vi "main 0.9.5.testing.vi"() -> ()   [LabVIEW 2020]
uses:
  subvi/Newport ESP301/Newport ESP301.lvlib
  subvi/sp_manip.llb/sp_manip_lib.lvlib
  subvi/sp_manip.llb/tcp_gateway.lvlib
  subvi/PHOIBOS/DEFINITIONS/DEF_dev_type.ctl
  subvi/PHOIBOS/DEFINITIONS/DEF_dev_state.ctl
  <vilib>/Utility/file.llb/Write Delimited Spreadsheet (DBL).vi
  <vilib>/Utility/file.llb/Read Delimited Spreadsheet (string).vi
  <vilib>/Analysis/NI_AALBase.lvlib
  <vilib>/Analysis/1siggen.llb/Ramp Pattern by Samples.vi
  <vilib>/DAQmx/create/channels.llb/DAQmx Create Channel (AI-Voltage-Basic).vi
  <vilib>/DAQmx/read.llb/DAQmx Read (Analog DBL 1Chan 1Samp).vi
panel:
  out "Pics L":i32
  out "Pics NL":i32
  out "Voltage":dbl format="%0.2f"
  out "sideimg 2":dbl[][](graph)
  in  "Frame trigger \n(High Performance and QE only)":u16
  in  "Operating mode\nHP & QE / HS & DiCam Pro":u32
  out "Waveform Chart":dbl(graph)
  out "G2 X":cluster{dbl[], "Ramp Pattern":dbl[]}(graph)={array[344 elements], "Ramp Pattern"=[5593.0, 5541.0, 5578.0, 5573.0, 5542.0, 5582.0, 5523.0, 5570.0, 5578.0, 5560.0, 5581.0, 5542.0, 5577.0, 5517.0, 5599.0, 5558.0, 5549.0, 5571.0, 5527.0, 5574.0, 5565.0, 5561.0, 5570.0, 5531.0, 5576.0, 5531.0, 5576.0, 5554.0, 5523.0, 5573.0, 5536.0, 5555.0, 5539.0, 5549.0, 5543.0, 5541.0, 5581.0, 5523.0, 5548.0, 5528.0, 5558.0, 5565.0, 5537.0, 5556.0, 5521.0, 5538.0, 5549.0, 5532.0, 5562.0, 5512.0, 5555.0, 5549.0, 5536.0, 5542.0, 5511.0, 5567.0, 5526.0, 5549.0, 5545.0, 5543.0, 5562.0, 5518.0, 5561.0, 5490.0, 5542.0, 5522.0, 5529.0, 5542.0, 5521.0, 5556.0, 5511.0, 5541.0, 5534.0, 5512.0, 5569.0, 5525.0, 5547.0, 5507.0, 5533.0, 5533.0, 5501.0, 5555.0, 5497.0, 5517.0, 5526.0, 5519.0, 5565.0, 5503.0, 5548.0, 5496.0, 5544.0, 5523.0, 5534.0, 5533.0, 5501.0, 5529.0, 5494.0, 5523.0, 5526.0, 5519.0, 5539.0, 5493.0, 5508.0, 5532.0, 5504.0, 5546.0, 5540.0, 5550.0, 5488.0, 5556.0, 5535.0, 5510.0, 5535.0, 5515.0, 5543.0, 5475.0, 5538.0, 5528.0, 5504.0, 5523.0, 5502.0, 5535.0, 5473.0, 5503.0, 5501.0, 5531.0, 5525.0, 5490.0, 5524.0, 5484.0, 5520.0, 5506.0, 5492.0, 5516.0, 5477.0, 5511.0, 5487.0, 5509.0, 5496.0, 5467.0, 5538.0, 5494.0, 5512.0, 5497.0, 5498.0, 5526.0, 5482.0, 5506.0, 5466.0, 5522.0, 5489.0, 5512.0, 5518.0, 5475.0, 5547.0, 5480.0, 5569.0, 5504.0, 5485.0, 5528.0, 5506.0, 5529.0, 5468.0, 5524.0, 5507.0, 5518.0, 5511.0, 5471.0, 5525.0, 5480.0, 5482.0, 5510.0, 5506.0, 5522.0, 5475.0, 5540.0, 5477.0, 5511.0, 5514.0, 5500.0, 5497.0, 5484.0, 5536.0, 5476.0, 5485.0, 5527.0, 5509.0, 5529.0, 5495.0, 5504.0, 5496.0, 5519.0, 5512.0, 5469.0, 5506.0, 5465.0, 5502.0, 5481.0, 5508.0, 5519.0, 5499.0, 5515.0, 5476.0, 5496.0, 5502.0, 5499.0, 5494.0, 5477.0, 5541.0, 5477.0, 5512.0, 5497.0, 5472.0, 5511.0, 5471.0, 5503.0, 5507.0, 5504.0, 5477.0, 5479.0, 5508.0, 5481.0, 5522.0, 5517.0, 5516.0, 5505.0, 5502.0, 5491.0, 5481.0, 5512.0, 5484.0, 5500.0, 5478.0, 5493.0, 5529.0, 5492.0, 5518.0, 5471.0, 5518.0, 5490.0, 5513.0, 5497.0, 5488.0, 5517.0, 5477.0, 5524.0, 5464.0, 5495.0, 5514.0, 5495.0, 5522.0, 5477.0, 5490.0, 5535.0, 5489.0, 5491.0, 5491.0, 5515.0, 5473.0, 5504.0, 5505.0, 5515.0, 5510.0, 5473.0, 5521.0, 5475.0, 5537.0, 5499.0, 5505.0, 5509.0, 5460.0, 5509.0, 5473.0, 5489.0, 5500.0, 5464.0, 5522.0, 5471.0, 5528.0, 5475.0, 5502.0, 5494.0, 5511.0, 5516.0, 5486.0, 5528.0, 5471.0, 5492.0, 5477.0, 5491.0, 5531.0, 5486.0, 5549.0, 5498.0, 5524.0, 5482.0, 5495.0, 5505.0, 5476.0, 5512.0, 5444.0, 5512.0, 5498.0, 5471.0, 5489.0, 5462.0, 5502.0, 5459.0, 5503.0, 5489.0, 5493.0, 5498.0, 5461.0, 5505.0, 5495.0, 5503.0, 5459.0, 5501.0, 5515.0, 5459.0, 5510.0, 5469.0, 5504.0, 5499.0, 5505.0, 5524.0, 5477.0, 5527.0, 5477.0, 5475.0, 5495.0, 5482.0, 5514.0, 5481.0, 5499.0, 5481.0, 5482.0, 5498.0, 5460.0, 5469.0, 5471.0, 5519.0, 5495.0, 5485.0]}
  in  "reset every n pics":bool
  in  "pics2avg":i32=50
  in  "abort acq.":bool
  out "G2 Y":cluster{dbl[], "Ramp Pattern":dbl[]}(graph)={[5738.0, 5692.0, 5562.0, 5630.0, 5633.0, 5616.0, 5523.0, 5622.0, 5406.0, 5598.0, 5416.0, 5403.0, 5579.0, 5325.0, 5504.0, 5402.0, 5538.0, 5568.0, 5460.0, 5494.0, 5367.0, 5597.0, 5434.0, 5448.0, 5339.0, 5434.0, 5460.0, 5482.0, 5646.0, 5720.0, 5704.0, 5628.0, 5672.0, 5511.0, 5420.0, 5539.0, 5543.0, 5421.0, 5486.0, 5508.0, 5537.0, 5586.0, 5460.0, 5547.0, 5433.0, 5488.0, 5552.0, 5538.0, 5528.0, 5482.0, 5406.0, 5458.0, 5644.0, 5485.0, 5443.0, 5485.0, 5385.0, 5413.0, 5472.0, 5571.0, 5640.0, 5602.0, 5462.0, 5477.0, 5408.0, 5396.0, 5445.0, 5638.0, 5383.0, 5571.0, 5372.0, 5519.0, 5426.0, 5462.0, 5481.0, 5626.0, 5326.0, 5458.0, 5471.0, 5366.0, 5394.0, 5363.0, 5551.0, 5596.0, 5452.0, 5470.0, 5600.0, 5533.0, 5573.0, 5544.0, 5671.0, 5595.0, 5423.0, 5550.0, 5557.0, 5416.0, 5404.0, 5478.0, 5448.0, 5512.0, 5505.0, 5575.0, 5434.0, 5436.0, 5600.0, 5487.0, 5607.0, 5463.0, 5606.0, 5540.0, 5521.0, 5581.0, 5472.0, 5555.0, 5576.0, 5612.0, 5529.0, 5473.0, 5454.0, 5455.0, 5500.0, 5650.0, 5451.0, 5445.0, 5423.0, 5376.0, 5389.0, 5491.0, 5536.0, 5525.0, 5440.0, 5707.0, 5414.0, 5532.0, 5400.0, 5668.0, 5706.0, 5515.0, 5431.0, 5400.0, 5439.0, 5471.0, 5627.0, 5691.0, 5569.0, 5718.0, 5614.0, 5523.0, 5436.0, 5432.0, 5419.0, 5516.0, 5469.0, 5467.0, 5530.0, 5598.0, 5501.0, 5476.0, 5457.0, 5460.0, 5606.0, 5456.0, 5429.0, 5586.0, 5504.0, 5546.0, 5516.0, 5466.0, 5650.0, 5593.0, 5605.0, 5515.0, 5414.0, 5623.0, 5581.0, 5651.0, 5574.0, 5519.0, 5672.0, 5621.0, 5496.0, 5382.0, 5496.0, 5620.0, 5542.0, 5422.0, 5492.0, 5515.0, 5549.0, 5402.0, 5472.0, 5547.0, 5515.0, 5641.0, 5451.0, 5667.0, 5622.0, 5511.0, 5506.0, 5608.0, 5647.0, 5584.0, 5714.0, 5490.0, 5534.0, 5463.0, 5566.0, 5573.0, 5570.0, 5582.0, 5613.0, 5504.0, 5550.0, 5594.0, 5576.0, 5677.0, 5675.0, 5681.0, 5681.0, 5434.0, 5434.0, 5405.0, 5473.0, 5522.0, 5427.0, 5533.0, 5582.0, 5427.0, 5529.0, 5548.0, 5341.0, 5521.0, 5539.0, 5435.0, 5457.0, 5511.0, 5406.0, 5412.0, 5620.0, 5609.0, 5609.0, 5469.0, 5577.0, 5661.0, 5673.0, 5518.0, 5463.0, 5562.0, 5723.0, 5719.0, 5487.0, 5485.0, 5683.0, 5501.0, 5604.0, 5328.0], "Ramp Pattern"=[0.0, 1.003921568627451, 2.007843137254902, 3.011764705882353, 4.015686274509804, 5.019607843137255, 6.023529411764706, 7.027450980392157, 8.031372549019608, 9.035294117647059, 10.03921568627451, 11.04313725490196, 12.047058823529412, 13.050980392156863, 14.054901960784314, 15.058823529411764, 16.062745098039215, 17.066666666666666, 18.070588235294117, 19.07450980392157, 20.07843137254902, 21.08235294117647, 22.08627450980392, 23.090196078431372, 24.094117647058823, 25.098039215686274, 26.101960784313725, 27.105882352941176, 28.109803921568627, 29.113725490196078, 30.11764705882353, 31.12156862745098, 32.12549019607843, 33.129411764705885, 34.13333333333333, 35.13725490196079, 36.141176470588235, 37.14509803921569, 38.14901960784314, 39.15294117647059, 40.15686274509804, 41.16078431372549, 42.16470588235294, 43.168627450980395, 44.17254901960784, 45.1764705882353, 46.180392156862744, 47.1843137254902, 48.188235294117646, 49.1921568627451, 50.19607843137255, 51.2, 52.20392156862745, 53.207843137254905, 54.21176470588235, 55.21568627450981, 56.219607843137254, 57.22352941176471, 58.227450980392156, 59.23137254901961, 60.23529411764706, 61.23921568627451, 62.24313725490196, 63.247058823529414, 64.25098039215686, 65.25490196078431, 66.25882352941177, 67.26274509803922, 68.26666666666667, 69.27058823529411, 70.27450980392157, 71.27843137254902, 72.28235294117647, 73.28627450980392, 74.29019607843138, 75.29411764705883, 76.29803921568627, 77.30196078431372, 78.30588235294118, 79.30980392156863, 80.31372549019608, 81.31764705882352, 82.32156862745099, 83.32549019607843, 84.32941176470588, 85.33333333333333, 86.33725490196079, 87.34117647058824, 88.34509803921569, 89.34901960784313, 90.3529411764706, 91.35686274509804, 92.36078431372549, 93.36470588235294, 94.3686274509804, 95.37254901960785, 96.37647058823529, 97.38039215686274, 98.3843137254902, 99.38823529411765, 100.3921568627451, 101.39607843137254, 102.4, 103.40392156862745, 104.4078431372549, 105.41176470588235, 106.41568627450981, 107.41960784313726, 108.4235294117647, 109.42745098039215, 110.43137254901961, 111.43529411764706, 112.43921568627451, 113.44313725490196, 114.44705882352942, 115.45098039215686, 116.45490196078431, 117.45882352941176, 118.46274509803922, 119.46666666666667, 120.47058823529412, 121.47450980392156, 122.47843137254903, 123.48235294117647, 124.48627450980392, 125.49019607843137, 126.49411764705883, 127.49803921568628, 128.50196078431372, 129.50588235294117, 130.50980392156862, 131.51372549019607, 132.51764705882354, 133.521568627451, 134.52549019607844, 135.52941176470588, 136.53333333333333, 137.53725490196078, 138.54117647058823, 139.54509803921567, 140.54901960784315, 141.5529411764706, 142.55686274509804, 143.5607843137255, 144.56470588235294, 145.5686274509804, 146.57254901960783, 147.57647058823528, 148.58039215686276, 149.5843137254902, 150.58823529411765, 151.5921568627451, 152.59607843137255, 153.6, 154.60392156862744, 155.6078431372549, 156.61176470588236, 157.6156862745098, 158.61960784313726, 159.6235294117647, 160.62745098039215, 161.6313725490196, 162.63529411764705, 163.6392156862745, 164.64313725490197, 165.64705882352942, 166.65098039215687, 167.65490196078431, 168.65882352941176, 169.6627450980392, 170.66666666666666, 171.6705882352941, 172.67450980392158, 173.67843137254903, 174.68235294117648, 175.68627450980392, 176.69019607843137, 177.69411764705882, 178.69803921568626, 179.7019607843137, 180.7058823529412, 181.70980392156864, 182.71372549019608, 183.71764705882353, 184.72156862745098, 185.72549019607843, 186.72941176470587, 187.73333333333332, 188.7372549019608, 189.74117647058824, 190.7450980392157, 191.74901960784314, 192.75294117647059, 193.75686274509803, 194.76078431372548, 195.76470588235293, 196.7686274509804, 197.77254901960785, 198.7764705882353, 199.78039215686275, 200.7843137254902, 201.78823529411764, 202.7921568627451, 203.79607843137254, 204.8, 205.80392156862746, 206.8078431372549, 207.81176470588235, 208.8156862745098, 209.81960784313725, 210.8235294117647, 211.82745098039214, 212.83137254901962, 213.83529411764707, 214.8392156862745, 215.84313725490196, 216.8470588235294, 217.85098039215686, 218.8549019607843, 219.85882352941175, 220.86274509803923, 221.86666666666667, 222.87058823529412, 223.87450980392157, 224.87843137254902, 225.88235294117646, 226.8862745098039, 227.89019607843136, 228.89411764705883, 229.89803921568628, 230.90196078431373, 231.90588235294118, 232.90980392156862, 233.91372549019607, 234.91764705882352, 235.92156862745097, 236.92549019607844, 237.9294117647059, 238.93333333333334, 239.93725490196078, 240.94117647058823, 241.94509803921568, 242.94901960784313, 243.95294117647057, 244.95686274509805, 245.9607843137255, 246.96470588235294, 247.9686274509804, 248.97254901960784, 249.9764705882353, 250.98039215686273, 251.98431372549018, 252.98823529411766, 253.9921568627451, 254.99607843137255, 256.0]}
  out "ETA":timestamp=timestamp(3543843884.995538 s since 1904-01-01) format="%<%H:%M:%S>T"
  out "acq. imgs":i32=30
  out "snap_prog":dbl(slide)=1.0 scale=0.0..1.0
  in  "BasePath":path=path "Z:/PESdata"
  in  "cam_liveavg":bool caption="live average"
  out "cam_fps":dbl=20.079713544692744 caption="FPS" format="%.1g"
  out "sideimg":dbl[][](graph)
  in  "RunNumber":u16=77
  out "sum":dbl=4126991.0 format="%#.2g"
  out "max":dbl=54.0
  out "mainimg":dbl[][](graph)
  out "ESP_con?":bool=TRUE caption="ESP301"
  out "phoib_con?":bool caption="PHOIBOS"
  out "manip_con?":bool caption="manipulator"
  out "cam_con?":bool caption="camera"
  in  "main_close":bool
  in  "Tab Control":T1(tab)
  in  "manip_deltas":dbl[](array[numeric])=[0.0, 0.0, 0.0, 0.0, 10.0, 0.0] caption="delta" format="%#.5g"
  in  "aq.mode":enum32{"Radio Selection 1", "Radio Selection 2"}(radio)=enum."Radio Selection 2"
  in  "dark avg":i32=100
  in  "averages":i32=30 caption="N"
  in  "ESP_delta":dbl caption="relative [mm]"
  in  "ESP_-":bool
  in  "ESP_+":bool
  in  "ESP_go":bool
  in  "ESP_dest_t":dbl=250.17307139859977 caption="[fs]"
  in  "ESP_dest":dbl=31.304 caption="[mm]"
  in  "ESP_set_t0":bool
  in  "phoib_I_6s":dbl=3200.0
  in  "phoib_I_5s":dbl=1650.0
  in  "phoib_I_4s":dbl=4.558
  in  "phoib_I_3s":dbl=-7.0
  in  "phoib_I_2s":dbl=20.0
  in  "phoib_I_1s":dbl=22.0
  in  "phoib_standby":bool
  in  "phoib_set":bool
  out "phoib_I_6":dbl caption="Screen Voltage"
  out "phoib_I_5":dbl caption="Detctor Voltage"
  out "phoib_I_4":dbl caption="Work Function"
  out "phoib_I_3":dbl caption="Coil Current"
  out "phoib_I_2":dbl caption="Pass Energy"
  out "phoib_I_1":dbl caption="Kinetic Energy"
  out "Saved Positions":string[][](table)=[["ertwertwert", "-2.299945", "-2.030214", "38.900024", "50.000762", "0.000887", "-97.998082"], ["uztgugt", "-14.999451", "-13.638894", "442.380066", "13.998380", "-1.893758", "-76.305838"], ["asdf", "-14.999451", "-13.638894", "442.380066", "13.998380", "-1.893758", "-76.305838"], ["test3", "-14.999451", "-13.638894", "441.380066", "13.998380", "-1.893758", "-76.305838"]]
  in  "Save Pos":bool
  in  "Load":bool
  in  "Delete":bool
  in  "ManipRel +":bool
  in  "ManipRel -":bool
  in  "Move Abs":bool
  in  "stop manip":bool
  in  "dest":dbl[](array[numeric])=[-2.6172862113166087, -0.009888298846365134, 68.5008544921875, -46.36280498847848, 1.1073518432055398, -218.56360350415366] caption="destination" format="%#.5g"
  out "axis":string[](array[string])=["x", "y", "z", "polar", "tilt", "azimut"]
  out "pos":dbl[](array[numeric])=[-2.6172862113166087, -0.009888298846365134, 68.5008544921875, -46.363686276590336, 11.108982061941884, -218.56360350415366] caption="position" format="%.5f"
  in  "Mode":T2(ring)=enum."WideAngleMode"
  in  "VoltageRange":enum16{"3.5kV", "1.5kV", "400V", "100V", "10V"}(ring)=enum."400V"
  out "ESP_pos":dbl=31.4539 caption="Position"
  out "ESP_delay":dbl=1000.0251574040756 caption="Delay"
  out "ESP_t0":dbl=31.304 caption="Time Zero @"
  out "phoib_I_7":dbl caption="Conversion Voltage"
  in  "phoib_I_7s":dbl=-16.0
  in  "phoib_I_8s":dbl=0.0039
  in  "phoib_I_9s":dbl=0.0039
  out "phoib_I_8":dbl caption="FD1"
  out "phoib_I_9":dbl caption="FD2"
  in  "gain":bool
  in  "exposure [ms]":u32=1
  in  "binning":u16(ring)=2 items=["X 1", "X 2", "X 4", "X 8"]
  in  "cam_dark?":bool caption="subtract dark?"
  in  "cam_dark":bool
  in  "cam_saveimg":bool
  in  "e-size":u8
  in  "lower threshold":i32=-100
  in  "count?":bool
  in  "ROI Left":i32=1
  in  "ROI Right":i32=43
  in  "ROI Top":i32=1
  in  "ROI Bottom":i32=33
  out "moving?":bool[](array[boolean])
  in  "delscan_abort 2":bool
  in  "delscan_go 2":bool
  in  "delscan_finishIteration 2":bool
  out "del_ETA":timestamp=timestamp(3543843871.185777 s since 1904-01-01) format="%<%H:%M:%S>T"
  out "time / step":dbl=2.792118032773336
  out "duration [HH:MM:SS]":dbl=55.62603882380894 format="%<%H:%M:%S>t"
  out "disk [MB]":dbl=11.613000000000001
  out "RAM [MB]":dbl=2.765
  out "total steps":dbl=20.0
  out "delaypoints":dbl=5.0
  in  "generate delay table":bool
  in  "load delay table":bool
  in  "delay table [fs]":string[][](table)=[["-1000.000000"], ["-500.000000"], ["0.000000"], ["500.000000"], ["1000.000000"]]
  in  "delscan_iters":u32=4 caption="iterations"
  out "scangraph":T3(graph)
  in  "delscan_abort":bool
  out "delscan_progress":u32(slide)=5 scale=0.0..5.0
  in  "delscan_go":bool
  out "delscan_pos":dbl=31.453896228999998 caption="stage pos [mm]"
  in  "delscan_end":dbl=1000.0 caption="end [fs]"
  in  "delscan_stepsize":dbl=500.0 caption="stepsize [fs]"
  in  "delscan_start":dbl=-1000.0 caption="start [fs]"
  out "iteration":i32=5
  in  "delscan_finishIteration":bool
  in  "manip_scan_steps":u32=3
  in  "Optimize":bool
  in  "manip_scan_delta":dbl[](array[numeric])=[0.0, 0.0, 0.0, 0.0, 1.0, 0.0] caption="delta" format="%#.5g"
  out "delscan_progress 2":u32(slide)=2 scale=0.0..3.0
  in  "abort":bool
  in  "dev_bench":bool
  out "x/y":dbl
  out "1/x":dbl
  in  "stop":bool
  out "voltage out":dbl
  in  "manip_init":bool
  in  "manip_release":bool
  in  "phoib_init":bool
  in  "phoib_release":bool
  in  "ESP_init":bool
  in  "ESP_release":bool
  in  "ESP301 VISA":refnum<visa-resource-name>="COM8"
  in  "board number":i32
  in  "cam_init":bool
  in  "cam_release":bool
  out "cam_error":errorcluster
  out "phoib_error":errorcluster
  out "state":T4 items=["Off"=-1, "Standby"=0, "On"=1]
  in  "ESP Axis":i32=1 min=1 max=3
  out "error out":errorcluster
  out "error out 2":errorcluster={"status"=TRUE, "code"=1, "source"="TCP Write in sp_manip_lib.lvlib:sp_manip_disconnect.vi->main 0.9.1.vi"}
  # "0 = sequential\n1 = simultaneous"
  # "0 = internal\n1 = external rising\n2 = external falling"
  # "camera"
  # "analyzer"
  # "manipulator"
  # "aquisition"
  # "delay stage"
  # "Position"
  # "Destination"
  # "X\nY\nZ\npolar\ntilt\nazimut"
  # "camera"
  # "phoibos"
  # "ESP301"
  # "manipulator"
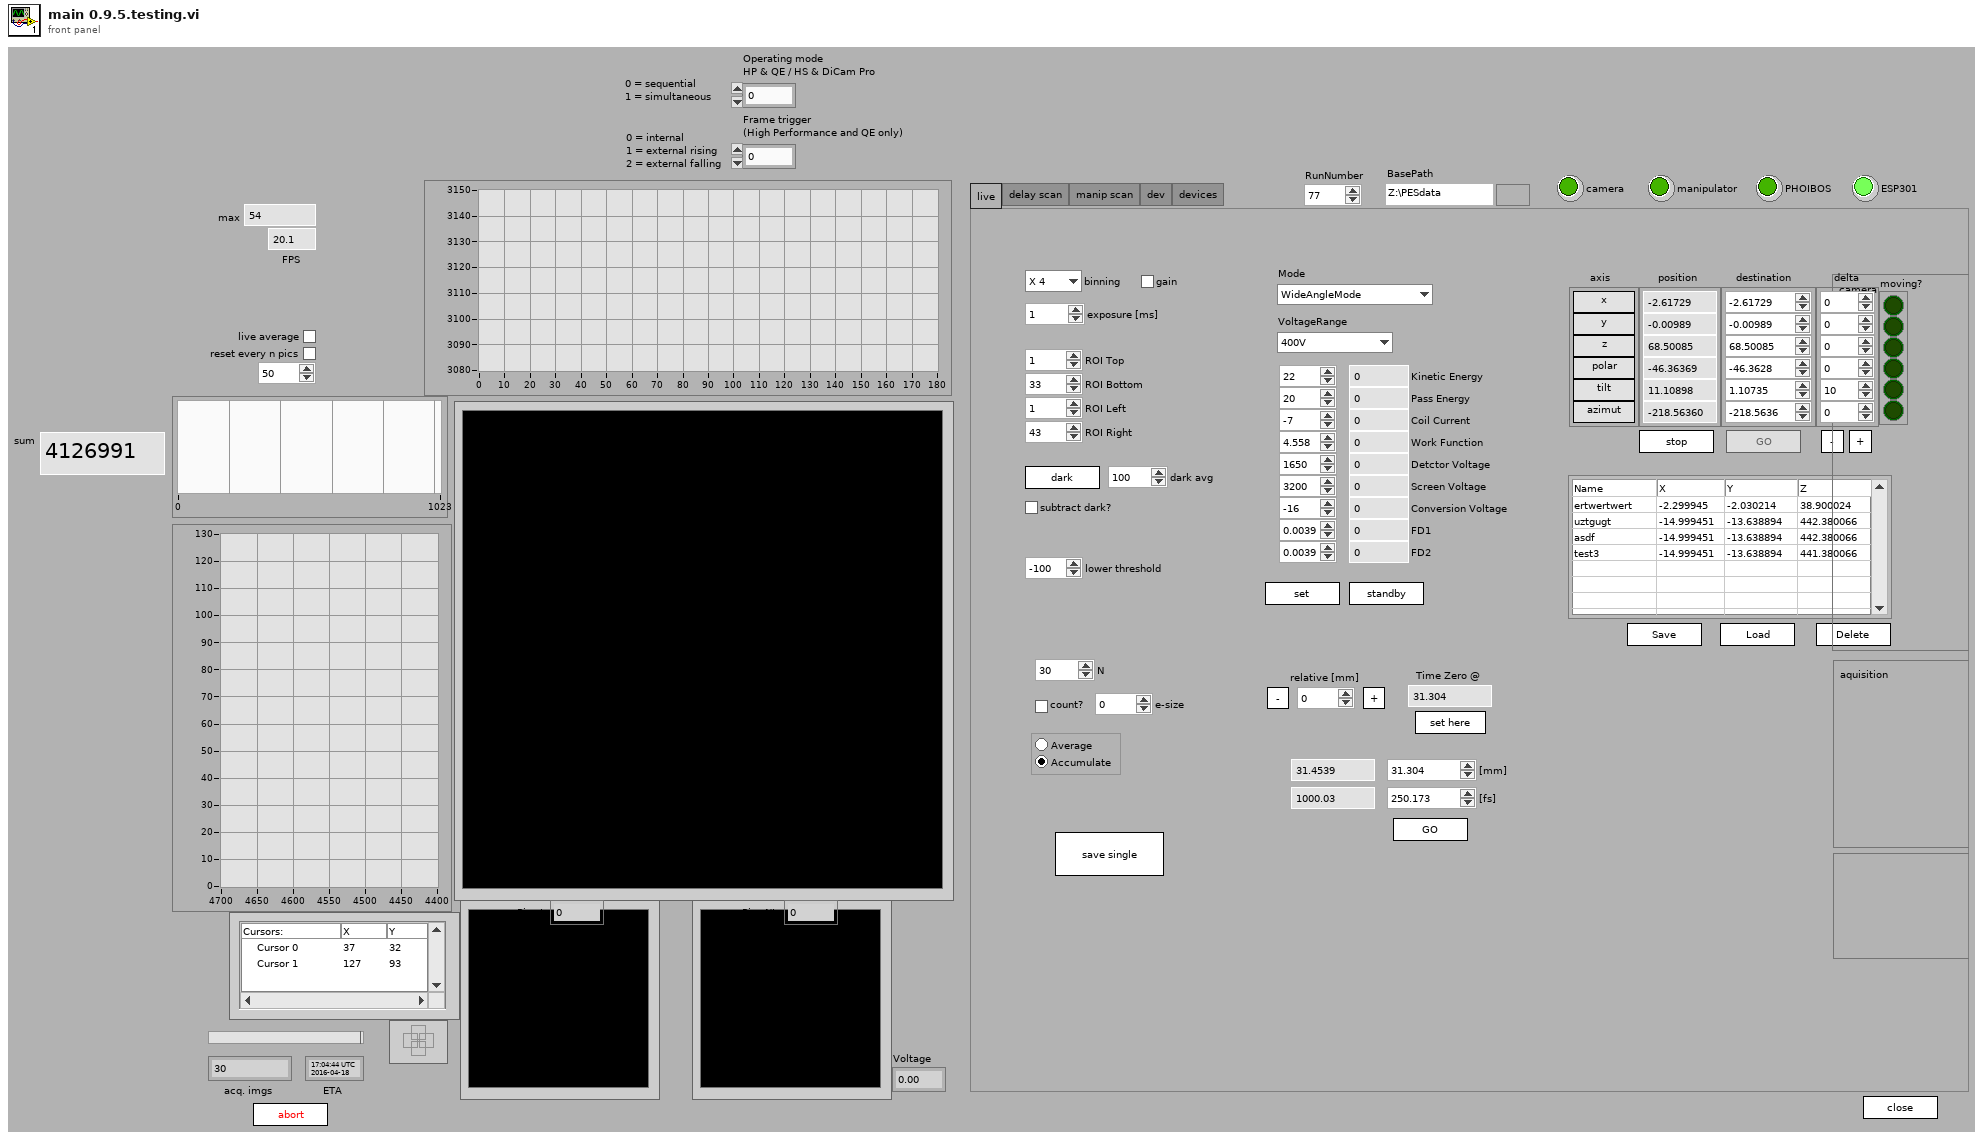
[diagram p1: front panel]
types:
  T1 = enum32{"live", "delay scan", "manip scan", "dev", "devices"}
  T2 = enum16{"HighMagnification", "MediumMagnification", "LowMagnification", "HighAngularDispersion", "MediumAngularDispersion", "LowAngularDispersion", "WideAngleMode", "LargeArea", "MediumArea", "SmallArea", "HighMagnification2", "SmallArea2", "ImagingMode"}
  T3 = cluster{"delay pointss [fs]":dbl[], "Intensity Chart":dbl[]}[]
  T4 = typedef "DEF_dev_state.ctl" = i32
  T5 = typedef "LVCursorListTypeDef.ctl" = cluster{"Name":string, "Color":u32, "Style":u8, "Point Style":u8, "Name Visible":bool, "Allow Drag":bool, "Cursor Mode":u32, "Plot":i32, "Index":i32, "Position":cluster{"X":dbl, "Y":dbl}, "X Scale":u32, "Y Scale":u32, "Watch Plots":i32[], "Watch All Plots":bool, "Plot Area":i32, "Label Offset":cluster{"X":dbl, "Y":dbl}}[]
  T6 = cluster{"delay pointss [fs]":dbl[], "Intensity Chart":dbl[]}
  T7 = cluster{"Camera type":u32, "Operating mode\nHP & QE / HS & DiCam Pro ":u32, "Frame trigger \n(High Performance and QE only)":u16, "Sequence trigger":u16, "Low Light\n(QE only)":bool, "Gain":bool, "Horzontal\nbinning":u16, "Vertical\nbinning ":u16, "ROI Left":i32, "ROI Right":i32, "ROI Top":i32, "ROI Bottom":i32}
  T8 = cluster{"Name":string, "Color":u32, "Style":u8, "Point Style":u8, "Name Visible":bool, "Allow Drag":bool, "Cursor Mode":u32, "Plot":i32, "Index":i32, "Position":cluster{"X":dbl, "Y":dbl}, "X Scale":u32, "Y Scale":u32, "Watch Plots":i32[], "Watch All Plots":bool, "Plot Area":i32, "Label Offset":cluster{"X":dbl, "Y":dbl}}
  T9 = cluster{"Axis_Name":string, "Axis_Type":string, "Axis_Position":dbl, "continous":bool, "moving":bool}[]
  T10 = typedef "DEF_dev_type.ctl" = enum32{"devA (analyzer)", "devD (detector)"}
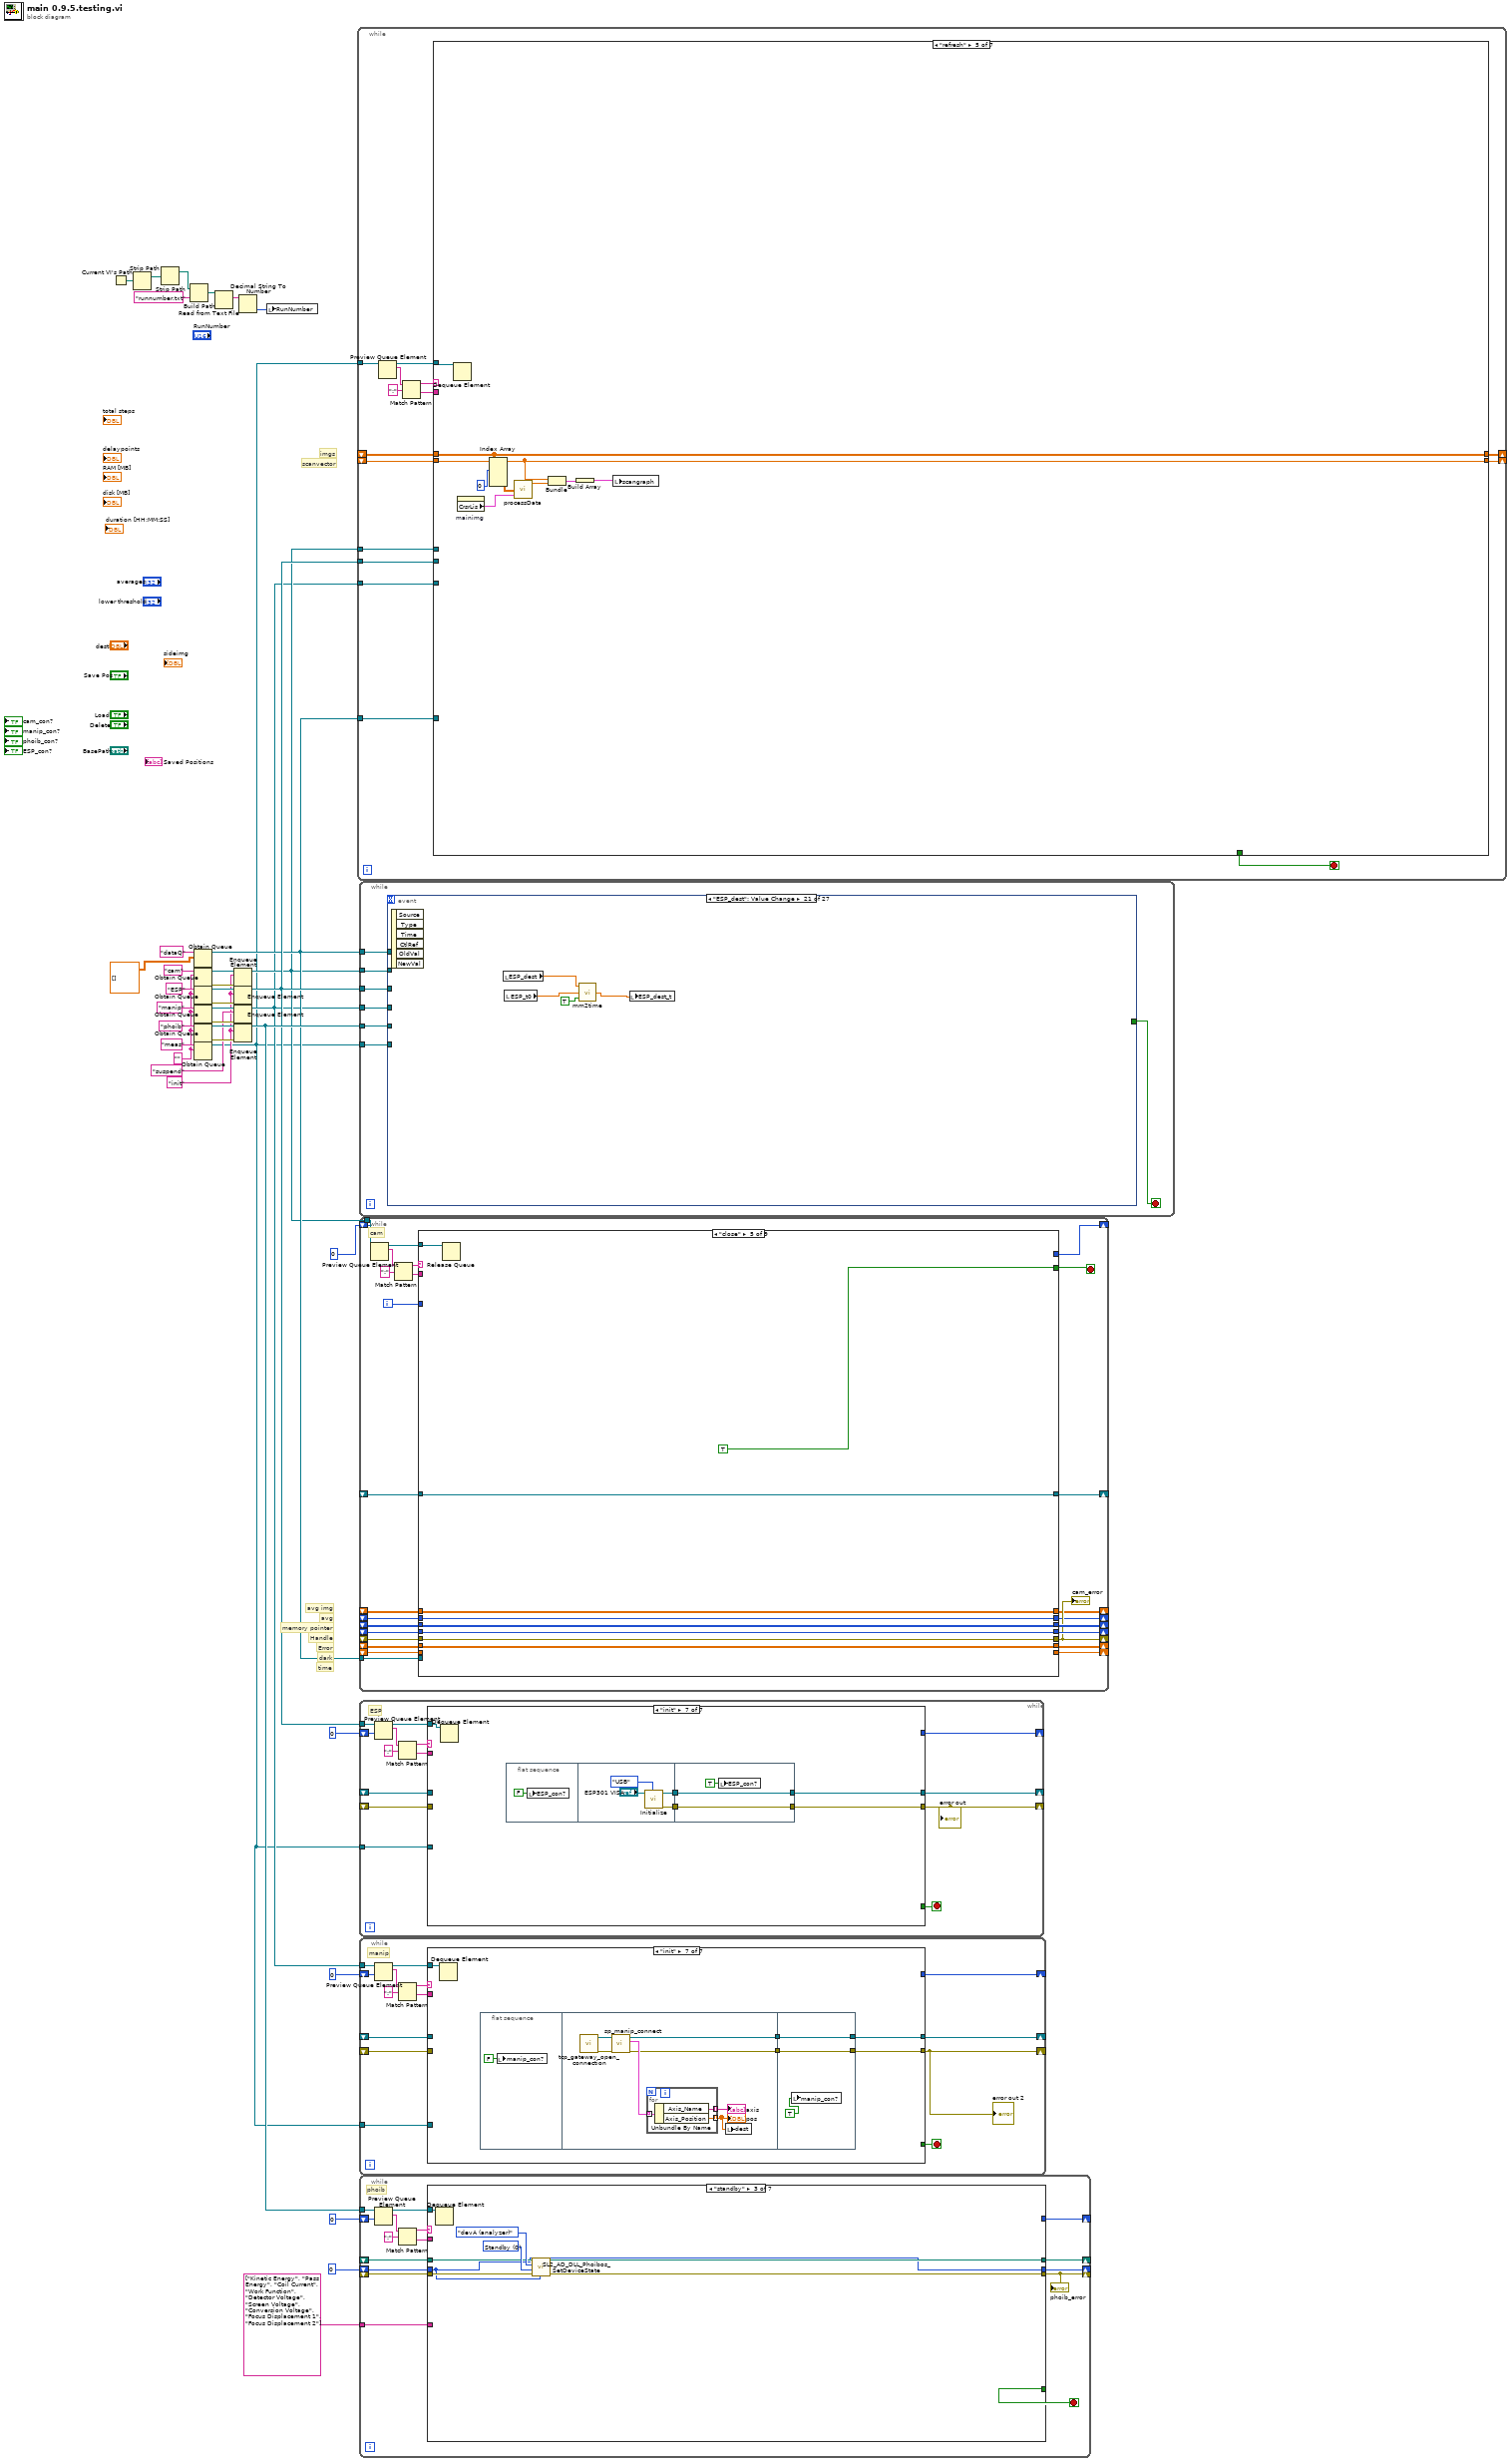
[diagram p0: block diagram]
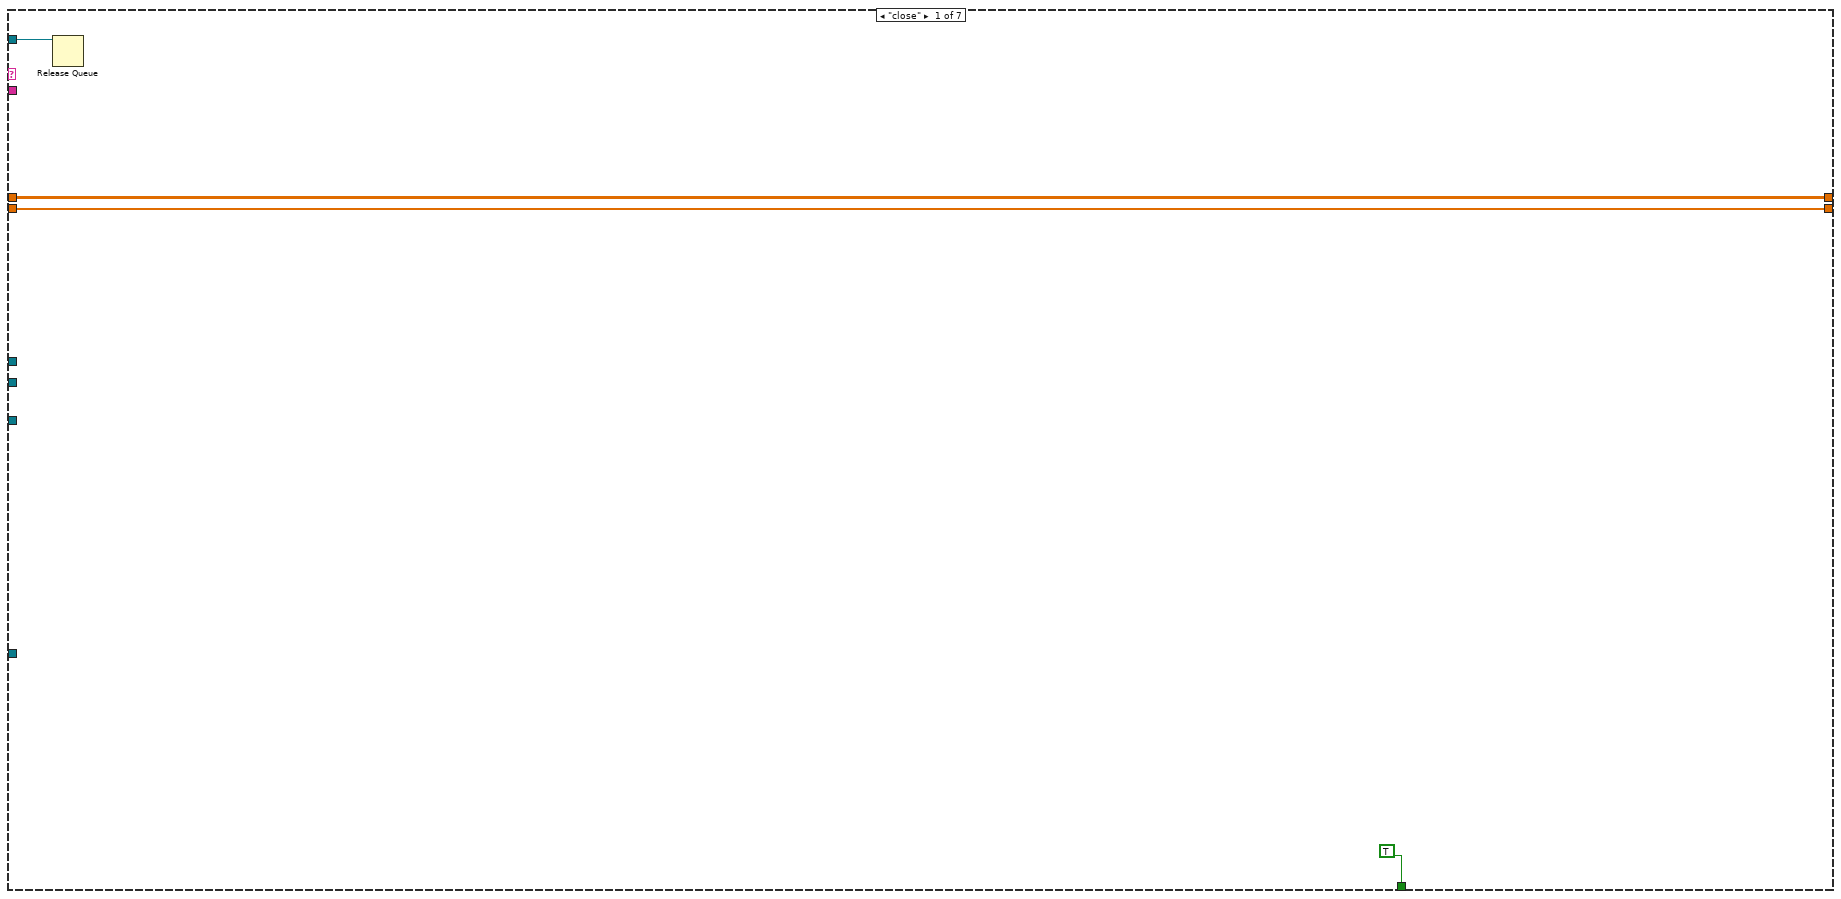
[diagram p2: hidden frame]
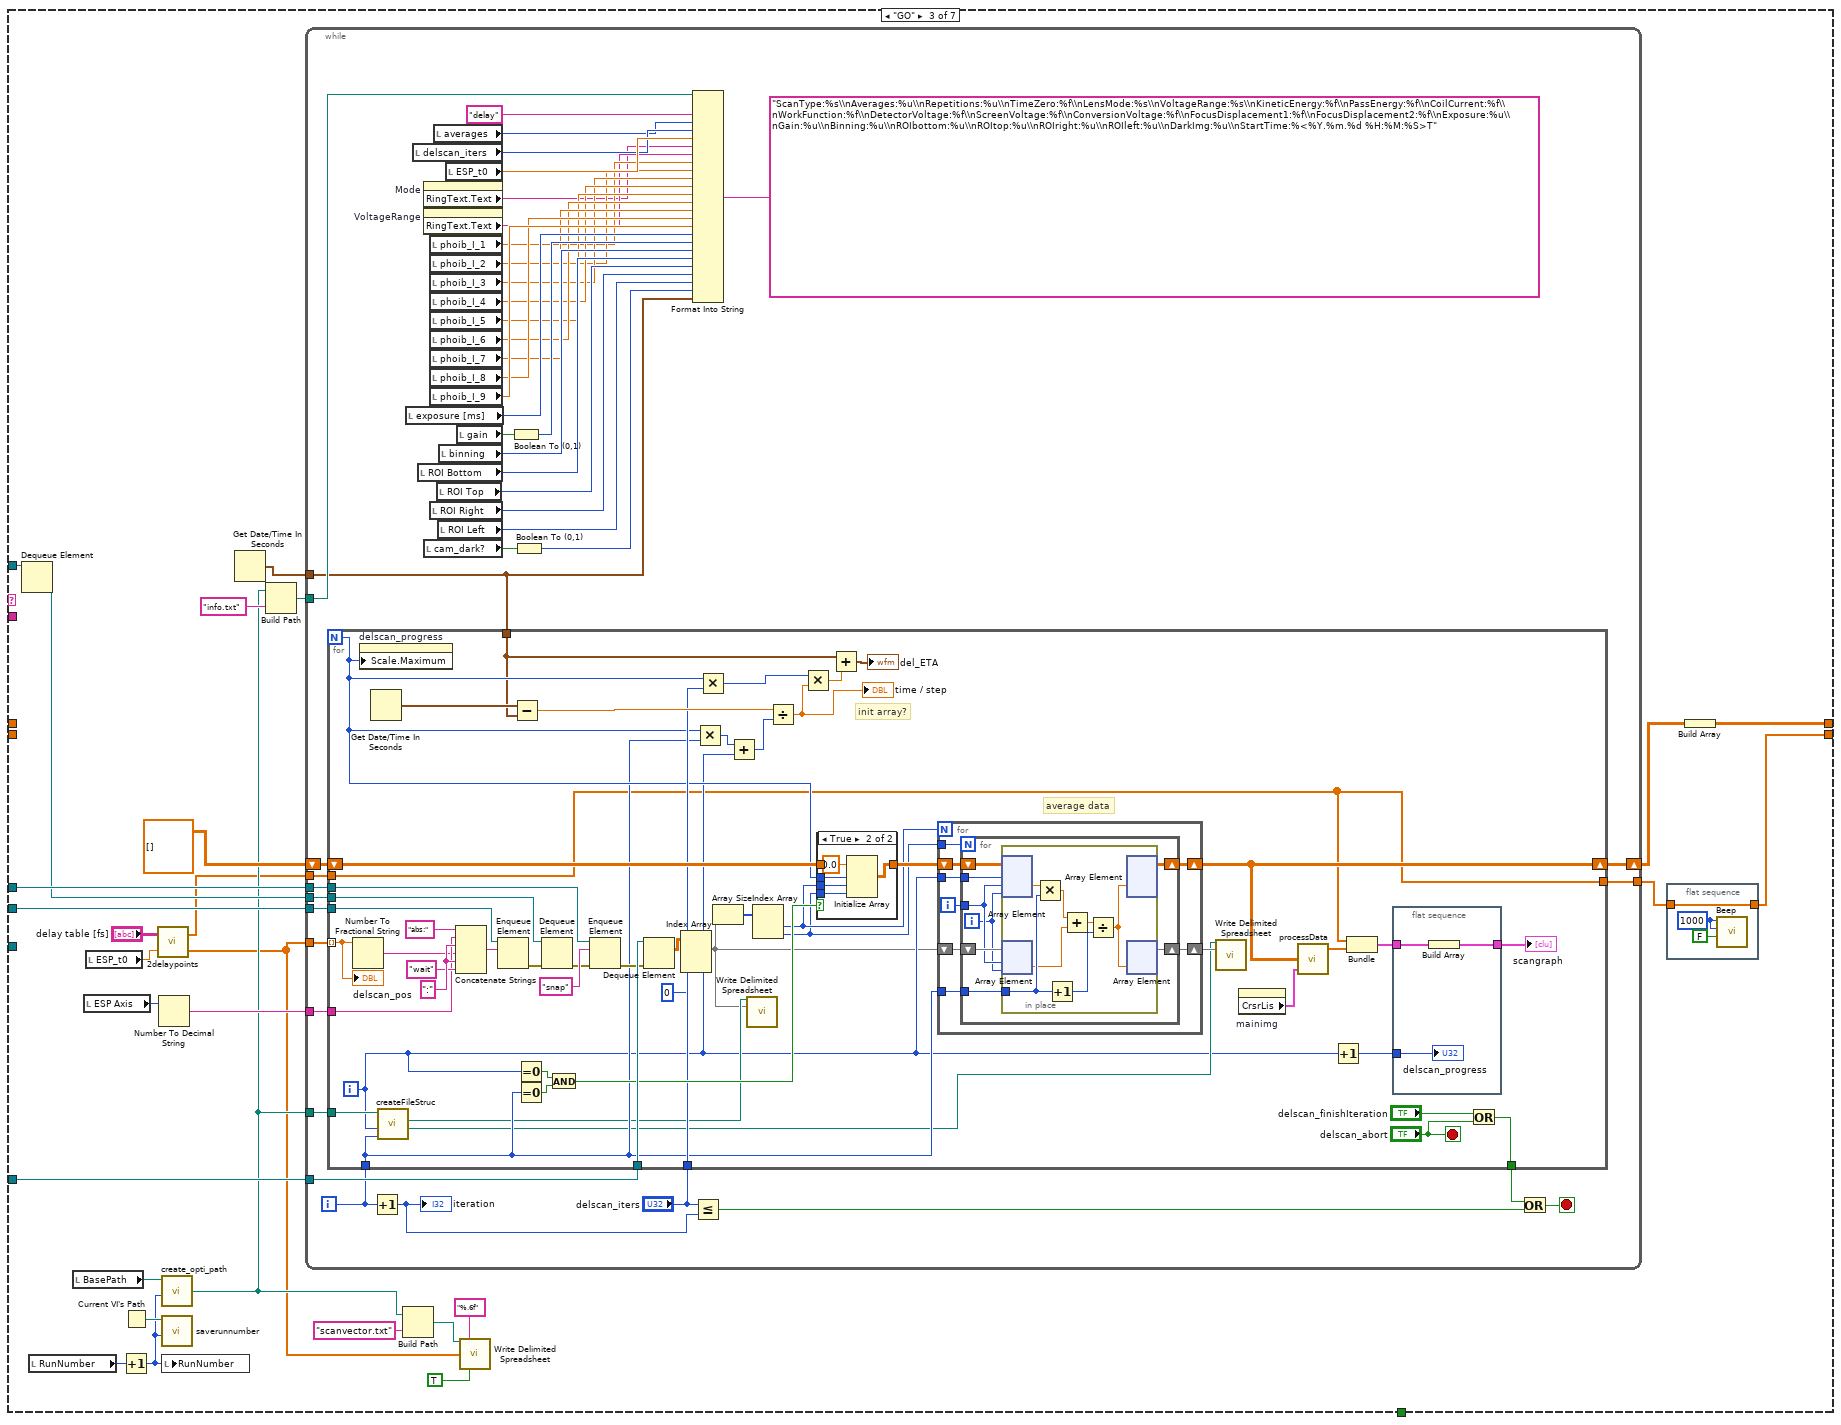
[diagram p4: hidden frame]
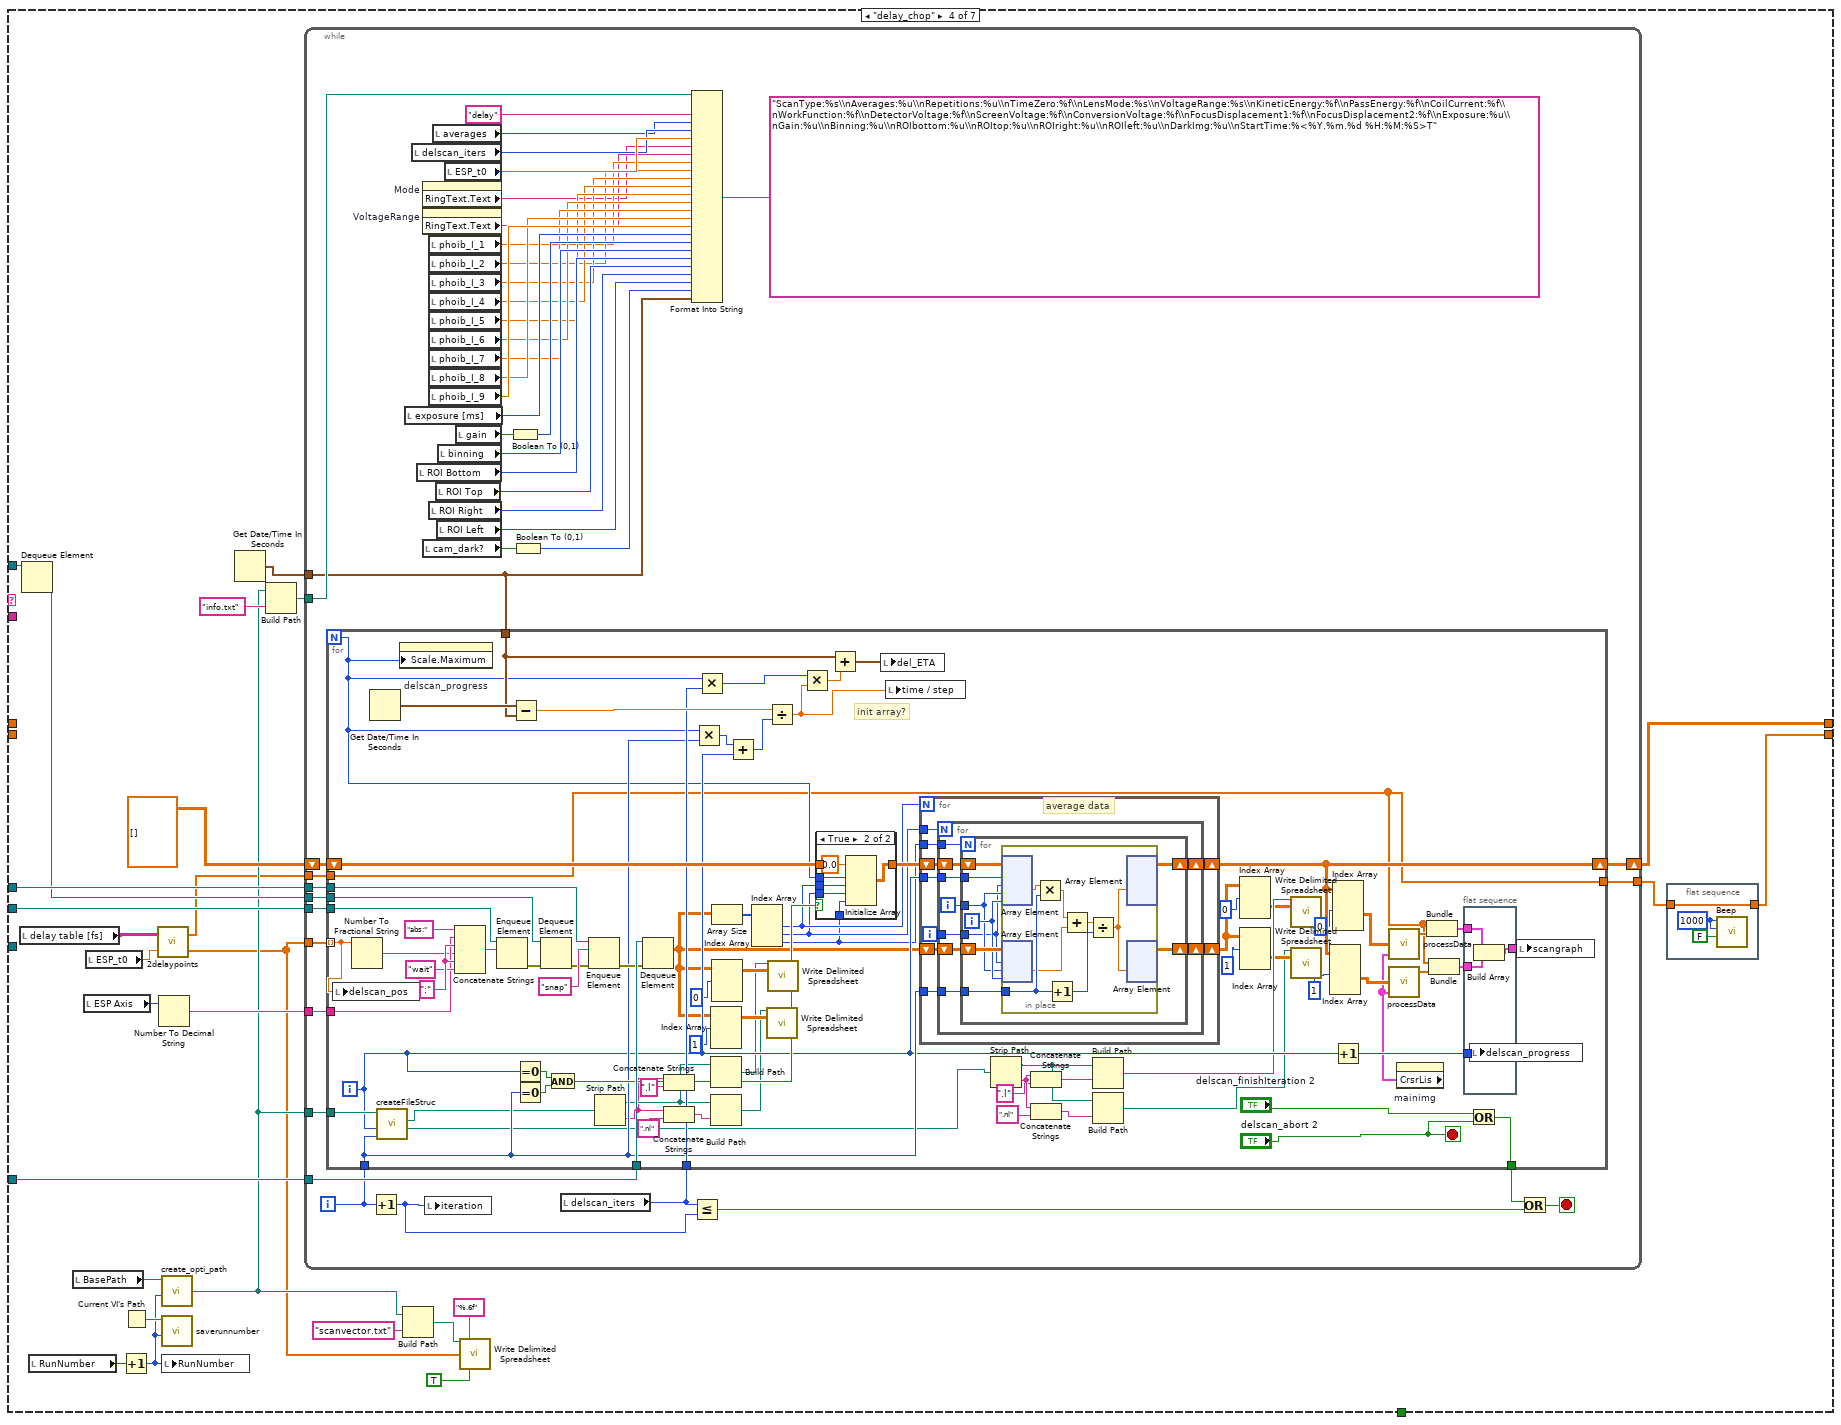
[diagram p6: hidden frame]
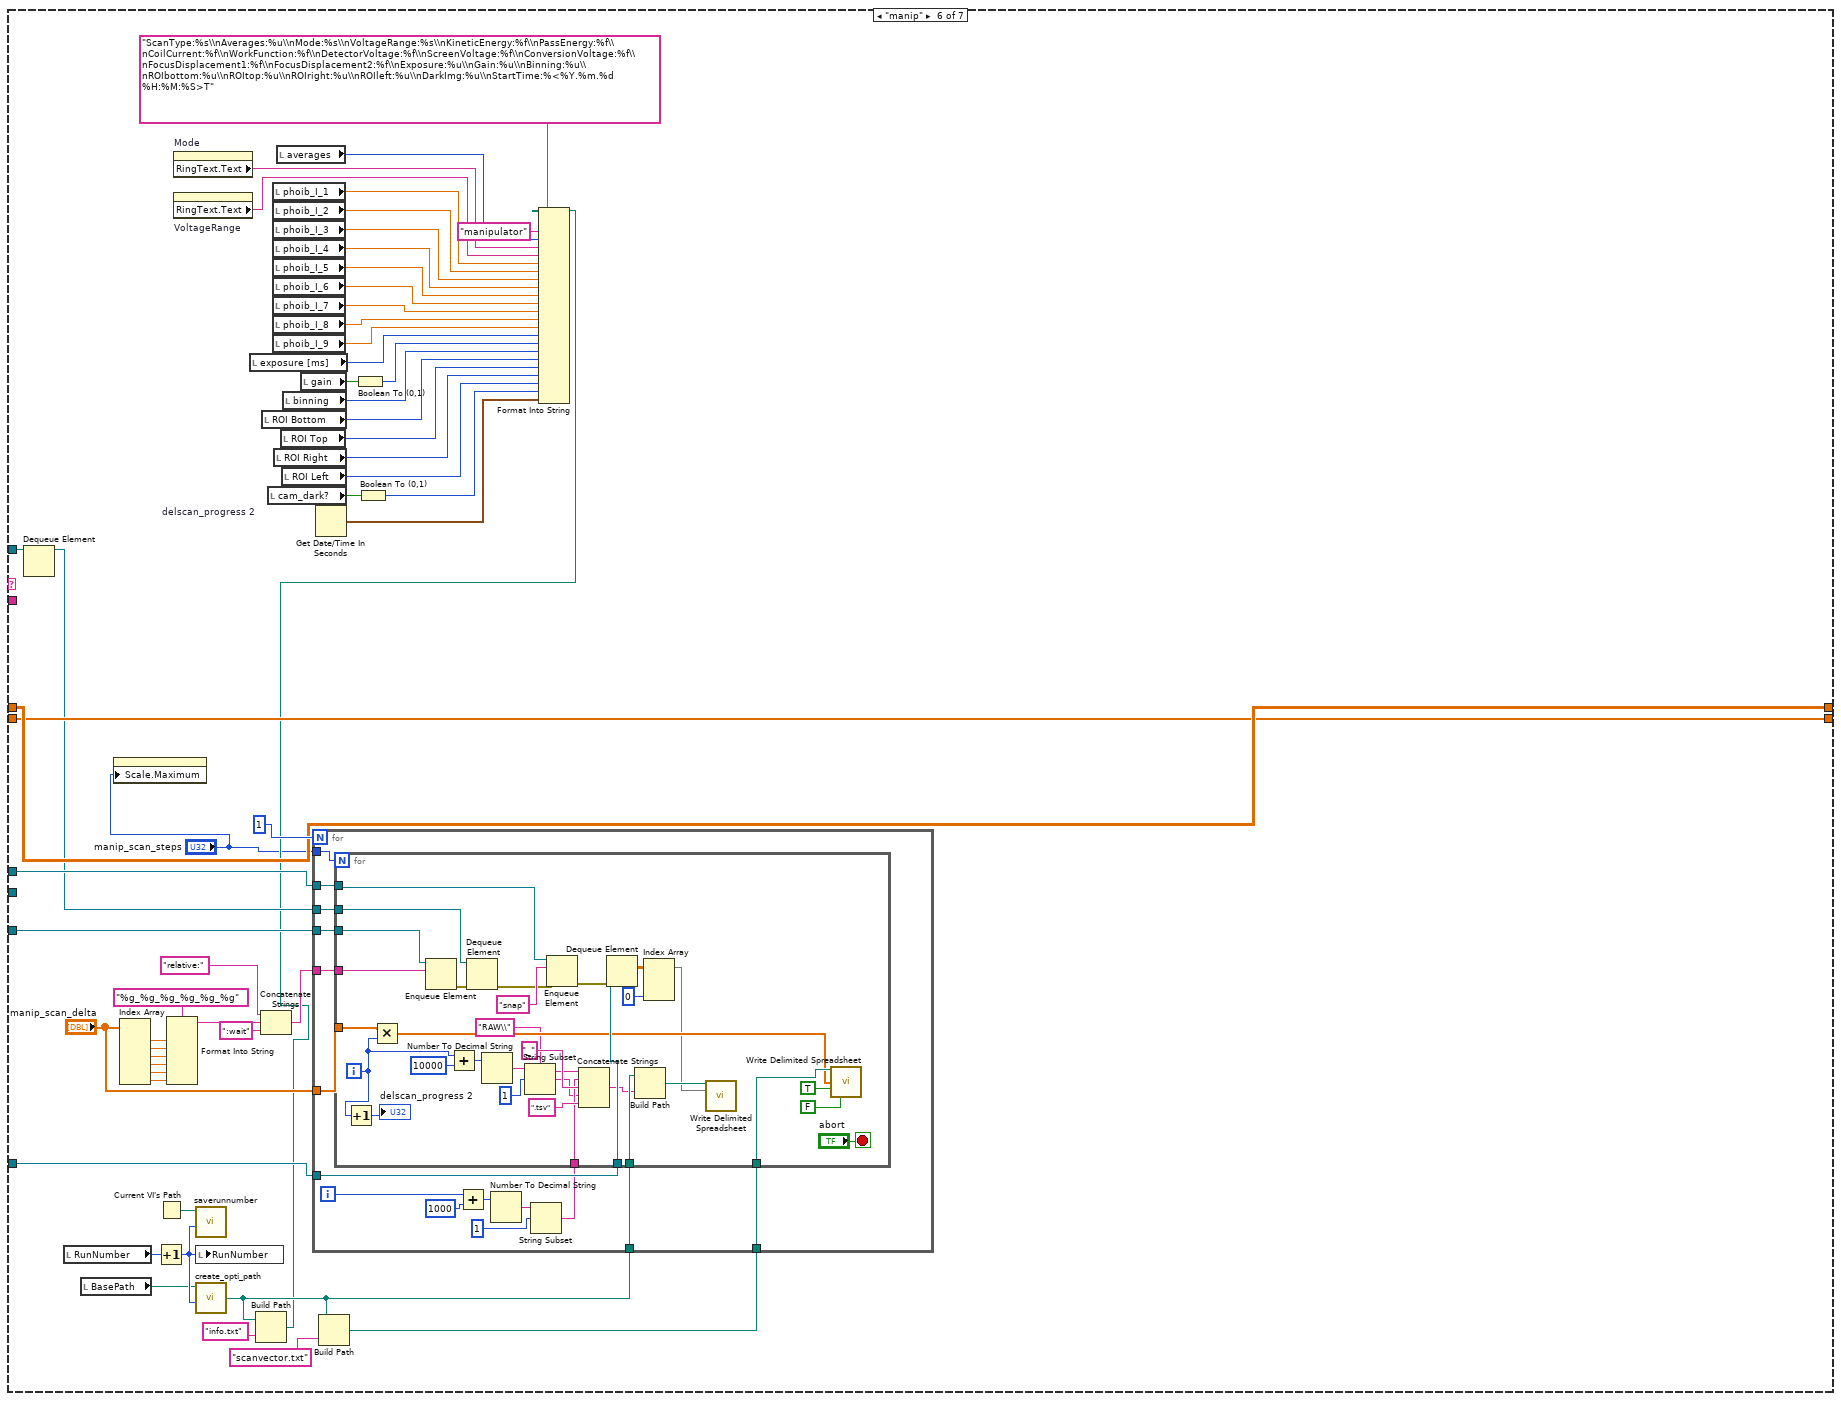
[diagram p8: hidden frame]
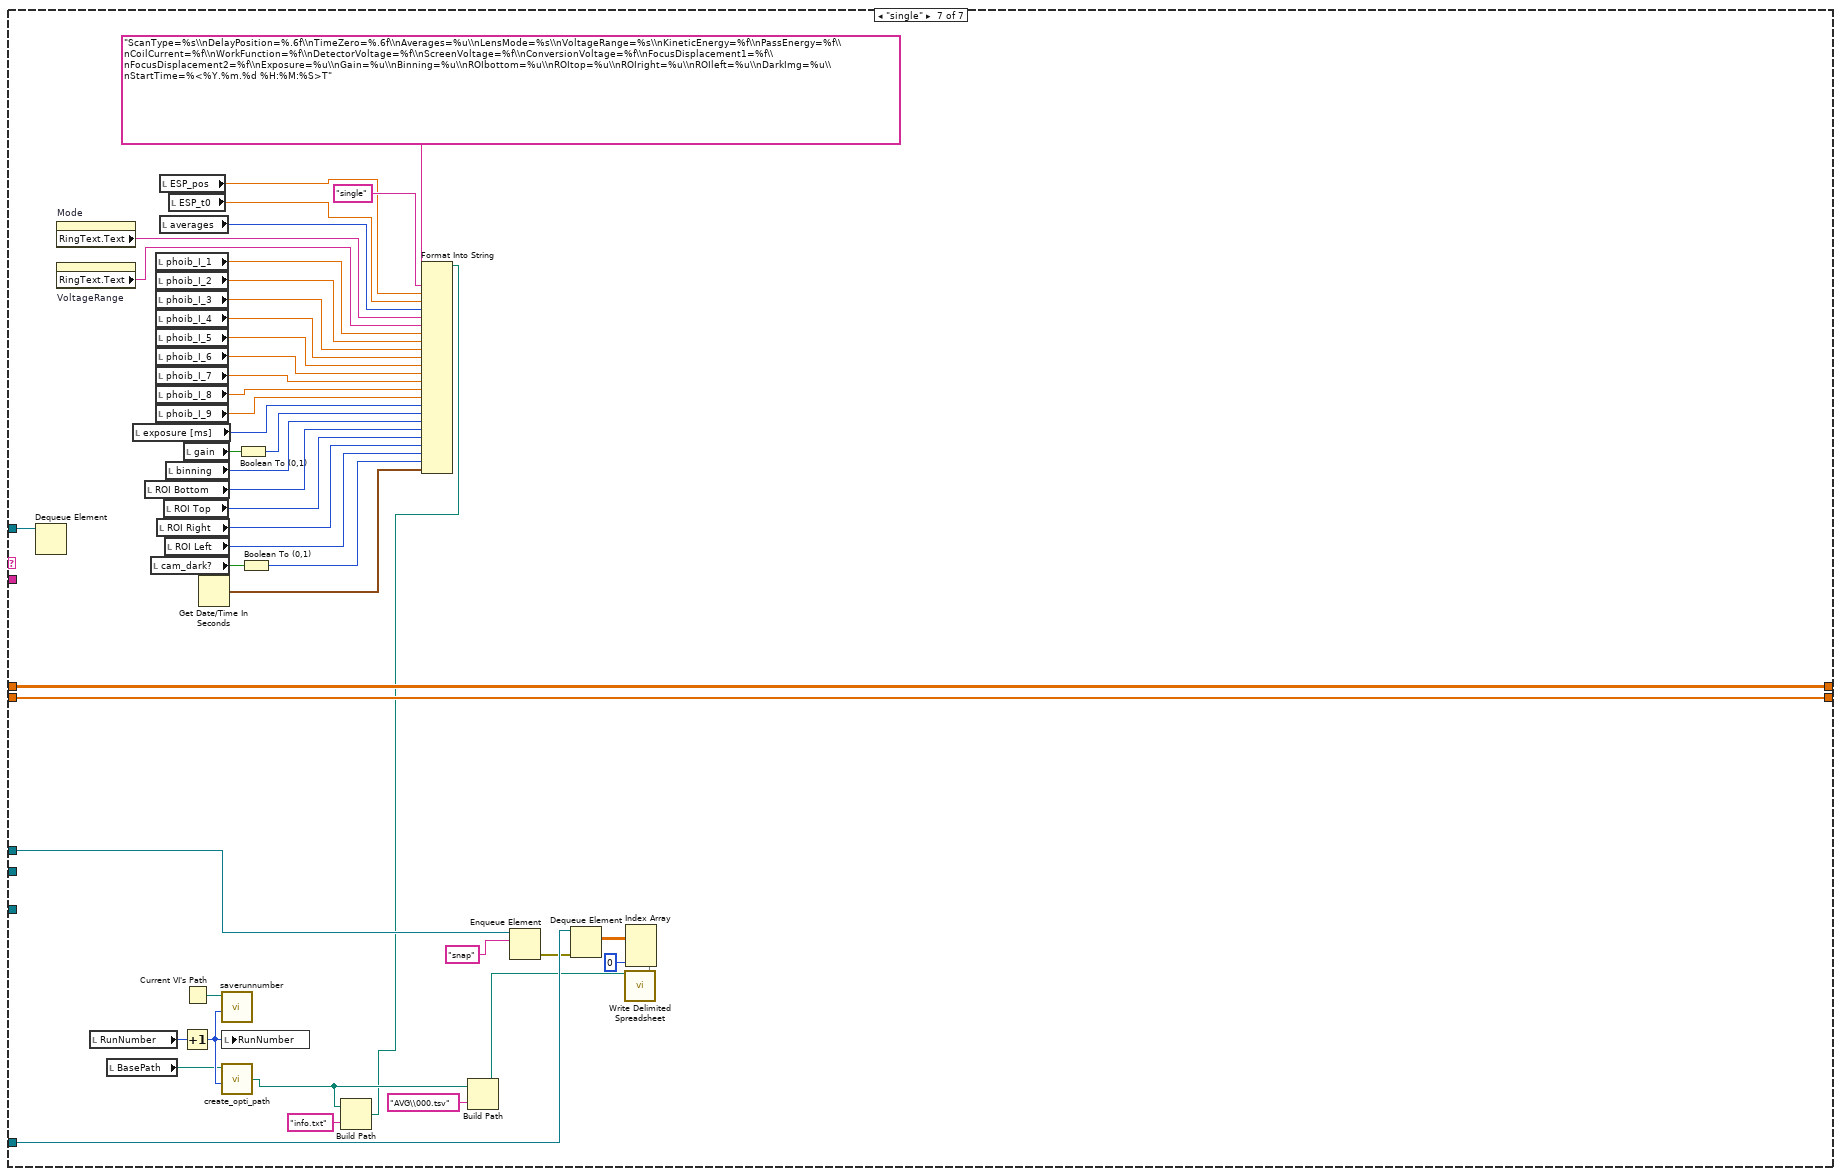
[diagram p9: hidden frame]
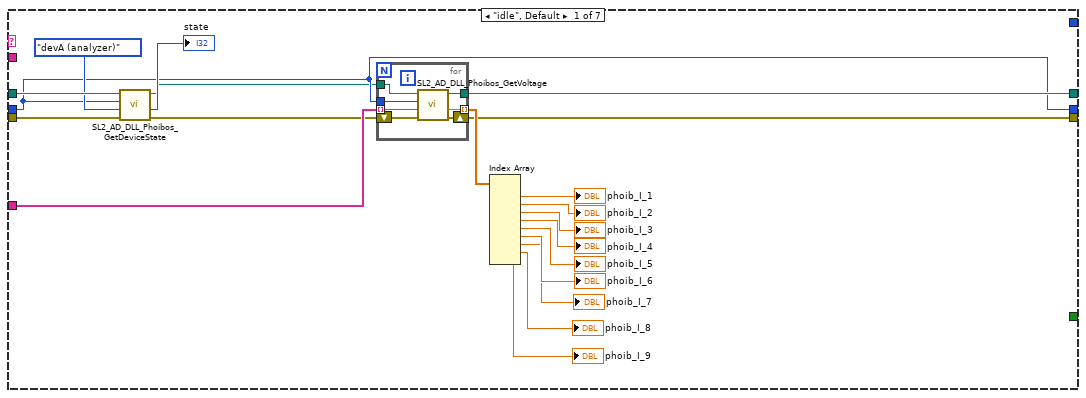
[diagram p10: hidden frame]
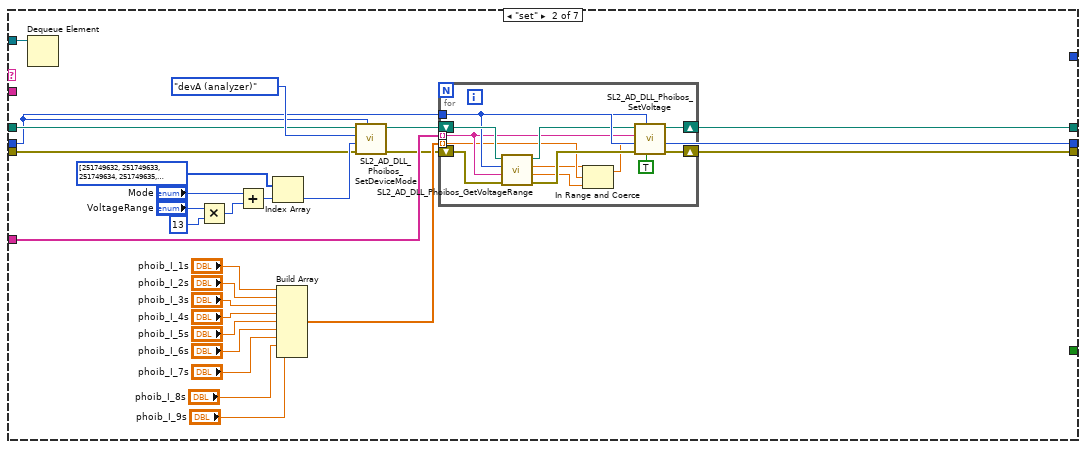
[diagram p11: hidden frame]
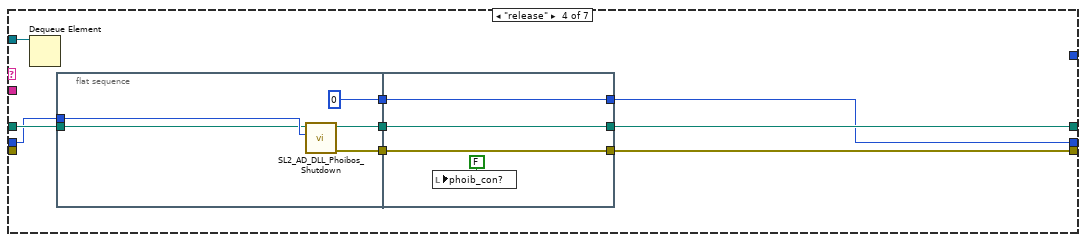
[diagram p12: hidden frame]
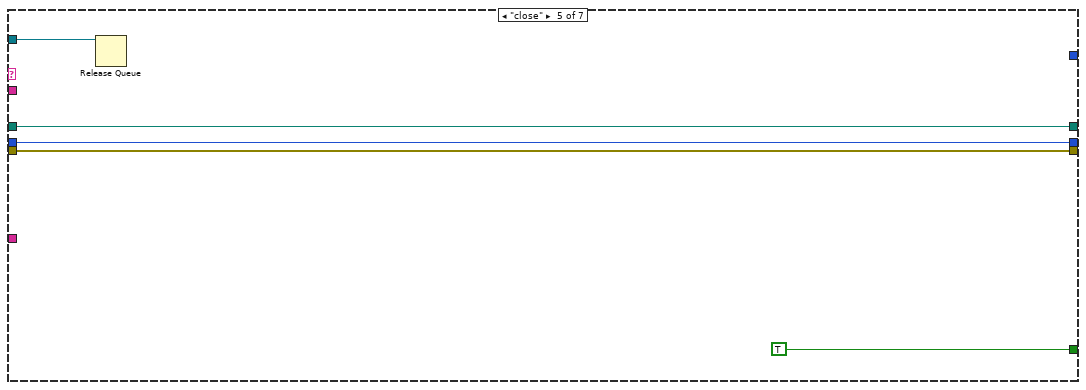
[diagram p13: hidden frame]
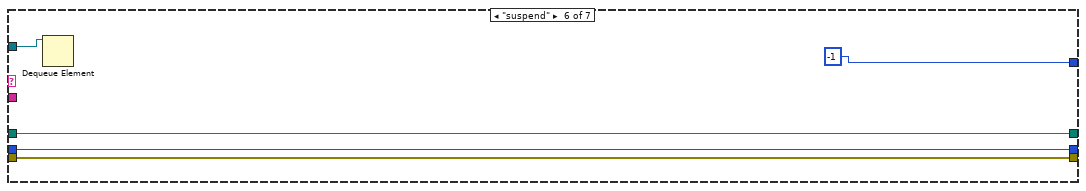
[diagram p14: hidden frame]
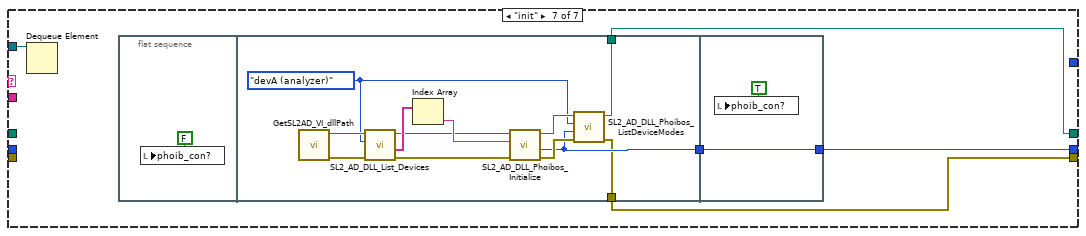
[diagram p15: hidden frame]
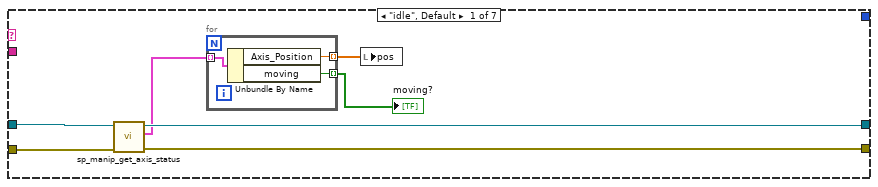
[diagram p16: hidden frame]
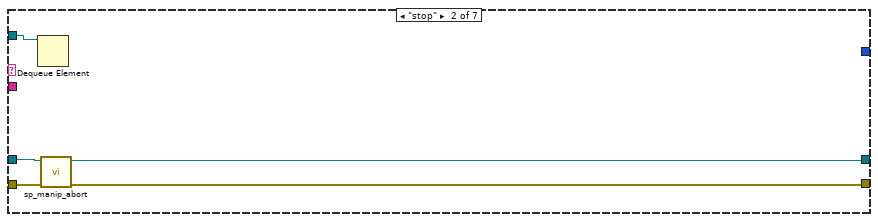
[diagram p17: hidden frame]
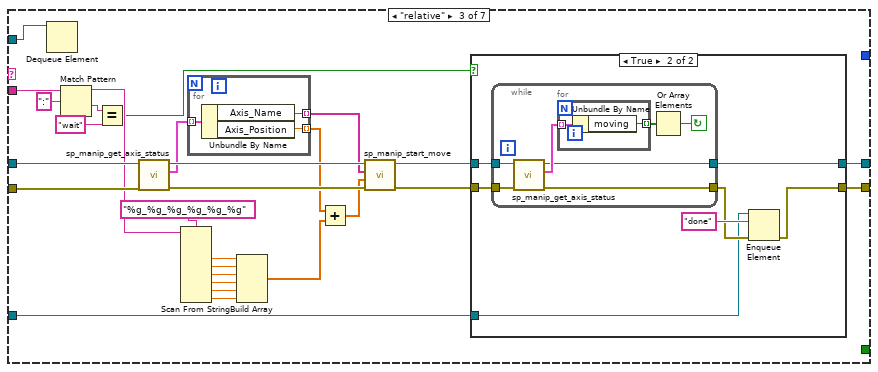
[diagram p18: hidden frame]
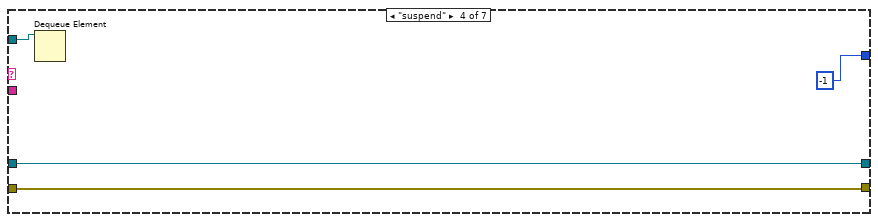
[diagram p20: hidden frame]
diagram:
  w14 = "init" ("name (unnamed)")
  w16 = "" ("name (unnamed)")
  # "scanvector"
  # "imgs"
  # "avg img"
  # "avg"
  # "time"
  # "dark"
  # "Error"
  # "Handle"
  # "memory pointer"
  n1 = Current VI's Path() -> (path=w4:path)
  n2 = Strip Path(path=w4) -> (stripped path=w8:path)  [unwired: 1 out]
  n3 = Strip Path(path=w8) -> (stripped path=w9:path)  [unwired: 1 out]
  n4 = Build Path(base path=w9, name or relative path="runnumber.txt") -> (appended path=w6:path)
  n5 = Obtain Queue(name (unnamed)="dataQ", element data type=dbl[][][] []) -> (queue out=w11:refnum<queue>)  [unwired: 3 in, 2 out]
  n6 = Obtain Queue(name (unnamed)="cam", element data type=w16) -> (queue out=w36:refnum<queue>, error out=w35:errorcluster)  [unwired: 3 in, 1 out]
  n7 = Obtain Queue(name (unnamed)="ESP", element data type=w16) -> (queue out=w33:refnum<queue>, error out=w34:errorcluster)  [unwired: 3 in, 1 out]
  n8 = Obtain Queue(name (unnamed)="manip", element data type=w16) -> (queue out=w30:refnum<queue>, error out=w29:errorcluster)  [unwired: 3 in, 1 out]
  n9 = Obtain Queue(name (unnamed)="phoib", element data type=w16) -> (queue out=w27:refnum<queue>, error out=w28:errorcluster)  [unwired: 3 in, 1 out]
  n10 = Obtain Queue(name (unnamed)="meas", element data type=w16) -> (queue out=w2:refnum<queue>)  [unwired: 3 in, 2 out]
  n11 = Read from Text File(file (use dialog)=w6) -> (text=w7:string)  [unwired: 3 in, 3 out]
  n12 = Enqueue Element(queue=w36, element=w14, error in (no error)=w35) -> (queue out=w10:refnum<queue>)  [unwired: 1 in, 2 out]
  n13 = Enqueue Element(queue=w33, element=w14, error in (no error)=w34) -> (queue out=w13:refnum<queue>)  [unwired: 1 in, 2 out]
  n14 = Enqueue Element(queue=w30, element="suspend" ("name (unnamed)"), error in (no error)=w29) -> (queue out=w3:refnum<queue>)  [unwired: 1 in, 2 out]
  n15 = Enqueue Element(queue=w27, element=w14, error in (no error)=w28) -> (queue out=w24:refnum<queue>)  [unwired: 1 in, 2 out]
  n16 = Decimal String To Number(string=w7) -> (number=w1:i32)  [unwired: 2 in, 1 out]
  n17 = local write "RunNumber"(w1) -> ()
  n18 = while {
    tunnel: w11 -> [w52]
    tunnel: w13 -> [w51]
    tunnel: w10 -> [w50]
    shift-right: [w47] -> _
    shift-left: _ -> [w49]
    shift-right: [w46] -> _
    shift-left: _ -> [w48]
    tunnel: w2 -> [w43]
    tunnel: w3 -> [w38]
    stop <- w39 stop-if-true
    n19 = Preview Queue Element(queue=w43) -> (queue out=w40:refnum<queue>, element=w45:string)  [unwired: 2 in, 2 out]
    n20 = Match Pattern(string=w45, regular expression=":") -> (before substring=w42:string, after substring=w41:string)  [unwired: 1 in, 2 out]
    n21 = case shown="\"refresh\"" w42 {
      tunnel: w52 -> [_ _ w86 w246 _ w467 w576]
      tunnel: w51 -> [_ _ w85 w245 _ _ _]
      tunnel: w50 -> [_ _ w84 w244 _ w466 w578]
      tunnel: w49 -> [w54 w58 _ _ w428 w463 w575]
      tunnel: w48 -> [w53 w57 _ _ w426 w462 w574]
      tunnel: [w54 w58 w59 w243 w428 w463 w575] -> w47
      tunnel: [w53 w57 w66 w226 w426 w462 w574] -> w46
      tunnel: w41 -> [_ _ _ _ _ _ _]
      tunnel: w40 -> [w56 _ w75 w235 w430 w461 w577]
      tunnel: [TRUE _ _ _ _ _ _] -> w39
      tunnel: w38 -> [_ _ _ _ _ w465 _]
      frame "close" {
        n22 = Release Queue(queue=w56) -> ()  [unwired: 2 in, 3 out]
      }
      frame "idle", Default {
      }
      frame "GO" {
        n23 = Dequeue Element(queue=w75) -> (queue out=w74:refnum<queue>)  [unwired: 2 in, 3 out]
        n24 = local read "RunNumber"() -> (w81:u16)
        n25 = local read "BasePath"() -> (w80:path)
        n26 = local read "ESP Axis"() -> (w78:i32)
        n27 = local read "ESP_t0"() -> (w64:dbl)
        n28 = Increment(x=w81) -> (x+1=w79:u16)
        n29 = Current VI's Path() -> (path=w82:path)
        n30 = call "2delaypoints.vi"("Offset (mm)"=w64, "delay table [fs]"="delay table [fs]") -> ("delay points [mm]"=w63:dbl[], "delay pointss [fs]"=w61:dbl[])
        n31 = Number To Decimal String(number=w78) -> (decimal integer string=w77:string)  [unwired: 1 in]
        n32 = call "create_opti_path.vi"("RunNumber"=w79, "base path"=w80) -> ("Path"=w71:path)  [unwired: 2 in]
        n33 = call "saverunnumber.vi"("RunNumber"=w79, "VI path"=w82) -> ()  [unwired: 10 in]
        n34 = local write "RunNumber"(w79) -> ()
        n35 = Get Date/Time In Seconds() -> (seconds since 1Jan1904=w60:timestamp)
        n36 = Build Path(base path=w71, name or relative path="info.txt") -> (appended path=w62:path)
        n37 = while {
          tunnel: w63 -> [w123]
          tunnel: w77 -> [w131]
          tunnel: w85 -> [w130]
          tunnel: w86 -> [w129]
          tunnel: w74 -> [w128]
          tunnel: w84 -> [w127]
          tunnel: w71 -> [w126]
          shift-right: [w124] -> w83
          shift-left: dbl[][][] [] -> [w125]
          tunnel: [w122] -> w67
          tunnel: w62 -> [w89]
          tunnel: w61 -> [w88]
          tunnel: w60 -> [w87]
          i -> [w121]
          stop <- w117 stop-if-true
          n38 = for {
            N -> [w153]
            tunnel: w123 -> [w162] mode=indexing
            tunnel: w131 -> [w179]
            tunnel: w130 -> [w178]
            tunnel: w129 -> [w173]
            tunnel: w128 -> [w177]
            tunnel: w127 -> [w176]
            tunnel: w126 -> [w147]
            shift-right: [w137] -> w124
            shift-left: w125 -> [w169]
            tunnel: w121 -> [w146]
            tunnel: w88 -> [w135]
            tunnel: [w135] -> w122
            tunnel: [w159] -> w119
            tunnel: w87 -> [w149]
            tunnel: "delscan_iters" -> [w154]
            i -> [w139]
            stop <- "delscan_abort" stop-if-true
            w181 = ":" ("string")
            # "average data"
            # "init array?"
            n39 = Number To Fractional String(number=w162) -> (F-format string=w171:string)  [unwired: 3 in]
            n40 = property on="delscan_progress" class="Slide (strict)"("Scale.Maximum"=w153) -> ()  [unwired: 2 in, 2 out]
            n41 = Get Date/Time In Seconds() -> (seconds since 1Jan1904=w157:timestamp)
            n42 = call "createFileStruc.vi"("i_iter"=w146, "i_delay"=w139, "meas_path"=w147) -> ("AVG file"=w142:path, "RAW file"=w143:path)  [unwired: 7 in]
            n43 = Concatenate Strings("abs:" ("string"), w179, w181, w171, w181, "wait" ("string")) -> (w184:string)
            n44 = Enqueue Element(queue=w178, element=w184) -> (error out=w182:errorcluster)  [unwired: 2 in, 2 out]
            n45 = Subtract(x=w157, y=w149) -> (x-y=w155:dbl)
            n46 = Equal To 0?(x=w139) -> (x = 0?=w145:bool)
            n47 = Equal To 0?(x=w146) -> (x = 0?=w144:bool)
            n48 = Dequeue Element(queue=w177, error in (no error)=w182) -> (error out=w174:errorcluster)  [unwired: 1 in, 3 out]
            n49 = And(x=w145, y=w144) -> (x .and. y?=w170:bool)
            n50 = Enqueue Element(queue=w176, element="snap", error in (no error)=w174) -> (error out=w172:errorcluster)  [unwired: 1 in, 2 out]
            n51 = Dequeue Element(queue=w173, error in (no error)=w172) -> (element=w165:dbl[][][])  [unwired: 1 in, 3 out]
            n52 = Index Array(array=w165, index (dim 2)=0 ("disabled index (col)")) -> (element=w133:dbl[][])  [unwired: 2 in]
            n53 = Multiply(x=w153, y=w146) -> (x*y=w158:i32)
            n54 = Multiply(x=w153, y=w154) -> (x*y=w152:u32)
            n55 = Array Size(array=w133) -> (size(s)=w166:i32[])
            n56 = Add(x=w158, y=w139) -> (x+y=w156:i32)
            n57 = call-poly <vilib>:"Write Delimited Spreadsheet.vi"("file path (dialog if empty)"=w143, "2D data"=w133) -> ()  [unwired: 12 in, 2 out]
            n58 = Index Array(array=w166) -> (element #1=w164:i32, element #2=w163:i32)  [unwired: 2 in]
            n59 = Divide(x=w155, y=w156) -> (x/y=w151:dbl)
            "time / step" <- w151
            n60 = Multiply(x=w152, y=w151) -> (x*y=w150:dbl)
            n61 = case shown="True" w170 {
              tunnel: w153 -> [_ w193]
              tunnel: [w188 w191] -> w168
              tunnel: w169 -> [w188 _]
              tunnel: w164 -> [_ w190]
              tunnel: w163 -> [_ w189]
              frame False {
              }
              frame True {
                n62 = Initialize Array(0.0 ("element"), w193, w190, w189) -> (w191:dbl[][][])
              }
            }
            n63 = Add(x=w149, y=w150) -> (x+y=→"del_ETA":timestamp)
            n64 = for {
              N: w164 -> [_]
              tunnel: w139 -> [w200]
              shift-right: [w198] -> w137
              shift-left: w168 -> [w201]
              tunnel: w146 -> [w196]
              shift-right: [w195] -> w167
              shift-left: w133 -> [w197]
              tunnel: w163 -> [w194]
              i -> [w199]
              n65 = for {
                N: w194 -> [_]
                tunnel: w200 -> [w208]
                tunnel: w199 -> [w205]
                shift-right: [w207] -> w198
                shift-left: w201 -> [w209]
                tunnel: w196 -> [w203]
                shift-right: [w202] -> w195
                shift-left: w197 -> [w206]
                i -> [w204]
                n66 = in-place {
                  in-place-border: w203 -> [w215]
                  n67 = in-place-array #1(w209, w208, w205, w204) -> (w216:dbl)
                  n68 = in-place-array #2(w206, w205, w204) -> (w213:dbl)
                  n69 = Multiply(x=w216, y=w215) -> (x*y=w214:dbl)
                  n70 = Increment(x=w215) -> (x+1=w211:i32)
                  n71 = Add(x=w214, y=w213) -> (x+y=w212:dbl)
                  n72 = Divide(x=w212, y=w211) -> (x/y=w210:dbl)
                  n73 = in-place-array #1(w210) -> (w207:dbl[][][])  [unwired: 3 out]
                  n74 = in-place-array #2(w210) -> (w202:dbl[][])  [unwired: 2 out]
                }
              }
            }
            n75 = call-poly <vilib>:"Write Delimited Spreadsheet.vi"("file path (dialog if empty)"=w142, "2D data"=w167) -> ()  [unwired: 12 in, 2 out]
            n76 = property on="mainimg" class="IntGraph (strict)"() -> ("CrsrLis"=w138:T5)  [unwired: 2 in, 2 out]
            n77 = call "processData.vi"("Cursor List"=w138, "data in"=w137) -> ("Intensity Chart"=w136:dbl[])  [unwired: 1 in, 2 out]
            n78 = Increment(x=w139) -> (x+1=w140:i32)
            n79 = Bundle("delay pointss [fs]"=w135, "Intensity Chart"=w136) -> (w134:T6)  [unwired: 1 in]
            n80 = flat-sequence {
              tunnel: w134 -> [w186]
              tunnel: [w185] -> w141
              tunnel: w140 -> [w187]
              frame #0 {
                n81 = Build Array(w186) -> (w185:T3)
                "delscan_progress" <- w187
              }
            }
            n82 = Or(x="delscan_finishIteration", y="delscan_abort") -> (x .or. y?=w159:bool)
            "delscan_pos" <- w162
            "scangraph" <- w141
          }
          n83 = Increment(x=w121) -> (x+1=w120:i32)
          "iteration" <- w120
          n84 = local read "exposure [ms]"() -> (w104:u32)
          n85 = local read "delscan_iters"() -> (w114:u32)
          n86 = local read "ROI Bottom"() -> (w107:i32)
          n87 = property on="Mode" class="Enum (strict)"() -> ("RingText.Text"=w93:string)  [unwired: 2 in, 2 out]
          n88 = property on="VoltageRange" class="Enum (strict)"() -> ("RingText.Text"=w94:string)  [unwired: 2 in, 2 out]
          n89 = local read "cam_dark?"() -> (w91:bool)
          n90 = local read "phoib_I_1"() -> (w95:dbl)
          n91 = local read "phoib_I_2"() -> (w96:dbl)
          n92 = local read "phoib_I_3"() -> (w97:dbl)
          n93 = local read "phoib_I_4"() -> (w98:dbl)
          n94 = local read "phoib_I_5"() -> (w99:dbl)
          n95 = local read "phoib_I_6"() -> (w100:dbl)
          n96 = local read "phoib_I_7"() -> (w101:dbl)
          n97 = local read "phoib_I_8"() -> (w102:dbl)
          n98 = local read "phoib_I_9"() -> (w103:dbl)
          n99 = local read "ROI Right"() -> (w109:i32)
          n100 = local read "averages"() -> (w113:i32)
          n101 = local read "ROI Top"() -> (w108:i32)
          n102 = local read "ROI Left"() -> (w110:i32)
          n103 = local read "binning"() -> (w106:u16)
          n104 = local read "ESP_t0"() -> (w115:dbl)
          n105 = local read "gain"() -> (w90:bool)
          n106 = Boolean To (0,1)(Boolean=w90) -> (0, 1=w105:i16)
          n107 = Boolean To (0,1)(Boolean=w91) -> (0, 1=w111:i16)
          n108 = Format Into String(format string="ScanType:%s\\nAverages:%u\\nRepetitions:%u\\nTimeZero:%f\\nLensMode:%s\\nVoltageRange:%s\\nKineticEnergy:%f\\nPassEnergy:%f\\nCoilCurrent:%f\\nWorkFunction:%f\\nDetectorVoltage:%f\\nScreenVoltage:%f\\nConversionVoltage:%f\\nFocusDisplacement1:%f\\nFocusDisplacement2:%f\\nExposure:%u\\nGain:%u\\nBinning:%u\\nROIbottom:%u\\nROItop:%u\\nROIright:%u\\nROIleft:%u\\nDarkImg:%u\\nStartTime:%<%Y.%m.%d %H:%M:%S>T", initial string=w89, "delay" ("input 1"), w113, w114, w115, w93, w94, w95, w96, w97, w98, w99, w100, w101, w102, w103, w104, w105, w106, w107, w108, w109, w110, w111, w87) -> ()  [unwired: 1 in, 2 out]
          n109 = Less Or Equal?(x="delscan_iters", y=w120) -> (x <= y?=w118:bool)
          n110 = Or(x=w119, y=w118) -> (x .or. y?=w117:bool)
        }
        n111 = Build Path(base path=w71, name or relative path="scanvector.txt") -> (appended path=w68:path)
        n112 = call-poly <vilib>:"Write Delimited Spreadsheet.vi"("file path (dialog if empty)"=w68, "format (%.3f)"="%.6f", "1D data"=w63, "transpose? (no:F)"=TRUE ("transpose? (F)")) -> ()  [unwired: 10 in, 2 out]
        n113 = flat-sequence {
          tunnel: w67 -> [w219]
          tunnel: [w219] -> w66
          frame #0 {
            w218 = u32 1000 ("frequency (Hz)")
            n114 = call <vilib>:"Beep.vi"("use system alert? (T)"=FALSE, "duration (msec)"=w218, "frequency (Hz)"=w218) -> ()  [unwired: 9 in]
          }
        }
        n115 = Build Array(w83) -> (w59:dbl[][][][])
      }
      frame "delay_chop" {
        n116 = local read "delay table [fs]"() -> (w220:string[][])
        n117 = Dequeue Element(queue=w235) -> (queue out=w234:refnum<queue>)  [unwired: 2 in, 3 out]
        n118 = local read "RunNumber"() -> (w241:u16)
        n119 = local read "BasePath"() -> (w240:path)
        n120 = local read "ESP Axis"() -> (w238:i32)
        n121 = local read "ESP_t0"() -> (w225:dbl)
        n122 = Increment(x=w241) -> (x+1=w239:u16)
        n123 = Current VI's Path() -> (path=w242:path)
        n124 = call "2delaypoints.vi"("Offset (mm)"=w225, "delay table [fs]"=w220) -> ("delay points [mm]"=w224:dbl[], "delay pointss [fs]"=w222:dbl[])
        n125 = Number To Decimal String(number=w238) -> (decimal integer string=w237:string)  [unwired: 1 in]
        n126 = call "create_opti_path.vi"("RunNumber"=w239, "base path"=w240) -> ("Path"=w231:path)  [unwired: 2 in]
        n127 = call "saverunnumber.vi"("RunNumber"=w239, "VI path"=w242) -> ()  [unwired: 10 in]
        n128 = local write "RunNumber"(w239) -> ()
        n129 = Get Date/Time In Seconds() -> (seconds since 1Jan1904=w221:timestamp)
        n130 = Build Path(base path=w231, name or relative path="info.txt") -> (appended path=w223:path)
        n131 = while {
          tunnel: w224 -> [w283]
          tunnel: w237 -> [w291]
          tunnel: w245 -> [w290]
          tunnel: w246 -> [w289]
          tunnel: w234 -> [w288]
          tunnel: w244 -> [w287]
          tunnel: w231 -> [w286]
          shift-right: [w284] -> w243
          shift-left: dbl[][][][] [] -> [w285]
          tunnel: [w282] -> w227
          tunnel: w223 -> [w251]
          tunnel: w222 -> [w250]
          tunnel: w221 -> [w249]
          i -> [w281]
          stop <- w278 stop-if-true
          n132 = Increment(x=w281) -> (x+1=w248:i32)
          n133 = local read "exposure [ms]"() -> (w266:u32)
          n134 = local read "delscan_iters"() -> (w276:u32)
          n135 = local read "ROI Bottom"() -> (w269:i32)
          n136 = property on="Mode" class="Enum (strict)"() -> ("RingText.Text"=w255:string)  [unwired: 2 in, 2 out]
          n137 = property on="VoltageRange" class="Enum (strict)"() -> ("RingText.Text"=w256:string)  [unwired: 2 in, 2 out]
          n138 = local read "cam_dark?"() -> (w253:bool)
          n139 = local write "iteration"(w248) -> ()
          n140 = local read "phoib_I_1"() -> (w257:dbl)
          n141 = local read "phoib_I_2"() -> (w258:dbl)
          n142 = local read "phoib_I_3"() -> (w259:dbl)
          n143 = local read "phoib_I_4"() -> (w260:dbl)
          n144 = local read "phoib_I_5"() -> (w261:dbl)
          n145 = local read "phoib_I_6"() -> (w262:dbl)
          n146 = local read "phoib_I_7"() -> (w263:dbl)
          n147 = local read "phoib_I_8"() -> (w264:dbl)
          n148 = local read "phoib_I_9"() -> (w265:dbl)
          n149 = local read "ROI Right"() -> (w271:i32)
          n150 = local read "averages"() -> (w275:i32)
          n151 = local read "ROI Top"() -> (w270:i32)
          n152 = local read "ROI Left"() -> (w272:i32)
          n153 = local read "binning"() -> (w268:u16)
          n154 = local read "ESP_t0"() -> (w277:dbl)
          n155 = local read "gain"() -> (w252:bool)
          n156 = Boolean To (0,1)(Boolean=w252) -> (0, 1=w267:i16)
          n157 = Boolean To (0,1)(Boolean=w253) -> (0, 1=w273:i16)
          n158 = local read "delscan_iters"() -> (w247:u32)
          n159 = for {
            N -> [w339]
            tunnel: w283 -> [w336] mode=indexing
            tunnel: w291 -> [w368]
            tunnel: w290 -> [w367]
            tunnel: w289 -> [w362]
            tunnel: w288 -> [w366]
            tunnel: w287 -> [w365]
            tunnel: w286 -> [w346]
            shift-right: [w322] -> w284
            shift-left: w285 -> [w358]
            tunnel: w281 -> [w345]
            tunnel: w250 -> [w319]
            tunnel: [w319] -> w282
            tunnel: [w355] -> w280
            tunnel: w249 -> [w347]
            tunnel: w247 -> [w350]
            i -> [w341]
            stop <- "delscan_abort 2" stop-if-true
            w370 = ":" ("string")
            # "init array?"
            n160 = local write "delscan_pos"(w336) -> ()
            n161 = Number To Fractional String(number=w336) -> (F-format string=w360:string)  [unwired: 3 in]
            n162 = Get Date/Time In Seconds() -> (seconds since 1Jan1904=w353:timestamp)
            n163 = call "createFileStruc.vi"("i_iter"=w345, "i_delay"=w341, "meas_path"=w346) -> ("AVG file"=w308:path, "RAW file"=w315:path)  [unwired: 7 in]
            n164 = property on="delscan_progress" class="Slide (strict)"("Scale.Maximum"=w339) -> ()  [unwired: 2 in, 2 out]
            n165 = Concatenate Strings("abs:" ("string"), w368, w370, w360, w370, "wait" ("string")) -> (w373:string)
            n166 = Enqueue Element(queue=w367, element=w373) -> (error out=w371:errorcluster)  [unwired: 2 in, 2 out]
            n167 = Subtract(x=w353, y=w347) -> (x-y=w351:dbl)
            n168 = Equal To 0?(x=w341) -> (x = 0?=w344:bool)
            n169 = Equal To 0?(x=w345) -> (x = 0?=w343:bool)
            n170 = Dequeue Element(queue=w366, error in (no error)=w371) -> (error out=w363:errorcluster)  [unwired: 1 in, 3 out]
            n171 = And(x=w344, y=w343) -> (x .and. y?=w359:bool)
            n172 = Enqueue Element(queue=w365, element="snap", error in (no error)=w363) -> (error out=w361:errorcluster)  [unwired: 1 in, 2 out]
            n173 = Strip Path(path=w315) -> (stripped path=w314:path, name=w311:string)
            n174 = Dequeue Element(queue=w362, error in (no error)=w361) -> (element=w331:dbl[][][])  [unwired: 1 in, 3 out]
            n175 = Concatenate Strings(w311, ".l" ("name or relative path")) -> (w309:string)
            n176 = Concatenate Strings(w311, ".nl" ("name or relative path")) -> (w312:string)
            n177 = Multiply(x=w339, y=w345) -> (x*y=w354:i32)
            n178 = Multiply(x=w339, y=w350) -> (x*y=w349:u32)
            n179 = Index Array(array=w331, index (dim 0)=1 ("disabled index (col)")) -> (element=w333:dbl[][])  [unwired: 2 in]
            n180 = Build Path(base path=w314, name or relative path=w309) -> (appended path=w330:path)
            n181 = Build Path(base path=w314, name or relative path=w312) -> (appended path=w329:path)
            n182 = Array Size(array=w331) -> (size(s)=w356:i32[])
            n183 = Index Array(array=w331, index (dim 0)=0 ("disabled index (col)")) -> (element=w332:dbl[][])  [unwired: 2 in]
            n184 = Add(x=w354, y=w341) -> (x+y=w352:i32)
            n185 = Index Array(array=w356) -> (element #1=w294:i32, element #2=w293:i32, element #3=w292:i32)  [unwired: 3 in]
            n186 = Divide(x=w351, y=w352) -> (x/y=w337:dbl)
            n187 = call-poly <vilib>:"Write Delimited Spreadsheet.vi"("file path (dialog if empty)"=w329, "2D data"=w333) -> ()  [unwired: 12 in, 2 out]
            n188 = call-poly <vilib>:"Write Delimited Spreadsheet.vi"("file path (dialog if empty)"=w330, "2D data"=w332) -> ()  [unwired: 12 in, 2 out]
            n189 = Multiply(x=w349, y=w337) -> (x*y=w348:dbl)
            n190 = case shown="True" w359 {
              tunnel: w339 -> [_ w418]
              tunnel: [w412 w416] -> w357
              tunnel: w358 -> [w412 _]
              tunnel: w294 -> [_ w415]
              tunnel: w293 -> [_ w414]
              tunnel: w292 -> [_ w413]
              frame False {
              }
              frame True {
                n191 = Initialize Array(0.0 ("element"), w418, w415, w414, w413) -> (w416:dbl[][][][])
              }
            }
            n192 = Add(x=w347, y=w348) -> (x+y=w338:timestamp)
            n193 = local write "del_ETA"(w338) -> ()
            n194 = local write "time / step"(w337) -> ()
            n195 = for {
              N: w294 -> [_]
              tunnel: w293 -> [w379]
              tunnel: w292 -> [w378]
              tunnel: w345 -> [w377]
              tunnel: w341 -> [w376]
              shift-right: [w375] -> w322
              shift-left: w357 -> [w382]
              shift-right: [w381] -> w326
              shift-left: w331 -> [w380]
              i -> [w374]
              # "average data"
              n196 = for {
                N: w379 -> [_]
                tunnel: w376 -> [w390]
                shift-right: [w388] -> w375
                shift-left: w382 -> [w391]
                tunnel: w377 -> [w386]
                shift-right: [w385] -> w381
                shift-left: w380 -> [w387]
                tunnel: w378 -> [w384]
                tunnel: w374 -> [w383]
                i -> [w389]
                n197 = for {
                  N: w384 -> [_]
                  tunnel: w390 -> [w393]
                  tunnel: w389 -> [w394]
                  shift-right: [w399] -> w388
                  shift-left: w391 -> [w400]
                  tunnel: w386 -> [w397]
                  shift-right: [w396] -> w385
                  shift-left: w387 -> [w398]
                  tunnel: w383 -> [w392]
                  i -> [w395]
                  n198 = in-place {
                    in-place-border: w397 -> [w406]
                    n199 = in-place-array #3(w400, w393, w392, w394, w395) -> (w407:dbl)
                    n200 = in-place-array #4(w398, w392, w394, w395) -> (w404:dbl)
                    n201 = Multiply(x=w407, y=w406) -> (x*y=w405:dbl)
                    n202 = Increment(x=w406) -> (x+1=w402:i32)
                    n203 = Add(x=w405, y=w404) -> (x+y=w403:dbl)
                    n204 = Divide(x=w403, y=w402) -> (x/y=w401:dbl)
                    n205 = in-place-array #3(w401) -> (w399:dbl[][][][])  [unwired: 4 out]
                    n206 = in-place-array #4(w401) -> (w396:dbl[][][])  [unwired: 3 out]
                  }
                }
              }
            }
            n207 = Strip Path(path=w308) -> (stripped path=w307:path, name=w306:string)
            n208 = Concatenate Strings(w306, ".l" ("name or relative path")) -> (w303:string)
            n209 = Concatenate Strings(w306, ".nl" ("name or relative path")) -> (w302:string)
            n210 = Build Path(base path=w307, name or relative path=w303) -> (appended path=w328:path)
            n211 = Build Path(base path=w307, name or relative path=w302) -> (appended path=w324:path)
            n212 = Index Array(array=w326, index (dim 0)=0 ("disabled index (col)")) -> (element=w327:dbl[][])  [unwired: 2 in]
            n213 = Index Array(array=w326, index (dim 0)=1 ("disabled index (col)")) -> (element=w325:dbl[][])  [unwired: 2 in]
            n214 = call-poly <vilib>:"Write Delimited Spreadsheet.vi"("file path (dialog if empty)"=w328, "2D data"=w327) -> ()  [unwired: 12 in, 2 out]
            n215 = call-poly <vilib>:"Write Delimited Spreadsheet.vi"("file path (dialog if empty)"=w324, "2D data"=w325) -> ()  [unwired: 12 in, 2 out]
            n216 = Index Array(array=w322, index (dim 1)=1 ("disabled index (col)")) -> (element=w321:dbl[][][])  [unwired: 3 in]
            n217 = Index Array(array=w322, index (dim 1)=0 ("disabled index (col)")) -> (element=w323:dbl[][][])  [unwired: 3 in]
            n218 = Increment(x=w341) -> (x+1=w342:i32)
            n219 = property on="mainimg" class="IntGraph (strict)"() -> ("CrsrLis"=w320:T5)  [unwired: 2 in, 2 out]
            n220 = call "processData.vi"("Cursor List"=w320, "data in"=w323) -> ("Intensity Chart"=w340:dbl[])  [unwired: 1 in, 2 out]
            n221 = call "processData.vi"("Cursor List"=w320, "data in"=w321) -> ("Intensity Chart"=w318:dbl[])  [unwired: 1 in, 2 out]
            n222 = Bundle("delay pointss [fs]"=w319, "Intensity Chart"=w340) -> (w317:T6)  [unwired: 1 in]
            n223 = Bundle("delay pointss [fs]"=w319, "Intensity Chart"=w318) -> (w316:T6)  [unwired: 1 in]
            n224 = flat-sequence {
              tunnel: w342 -> [w411]
              tunnel: w317 -> [w410]
              tunnel: w316 -> [w408]
              tunnel: [w409] -> w295
              frame #0 {
                n225 = local write "delscan_progress"(w411) -> ()
                n226 = Build Array(w410, w408) -> (w409:T3)
              }
            }
            n227 = Or(x="delscan_finishIteration 2", y="delscan_abort 2") -> (x .or. y?=w355:bool)
            n228 = local write "scangraph"(w295) -> ()
          }
          n229 = Format Into String(format string="ScanType:%s\\nAverages:%u\\nRepetitions:%u\\nTimeZero:%f\\nLensMode:%s\\nVoltageRange:%s\\nKineticEnergy:%f\\nPassEnergy:%f\\nCoilCurrent:%f\\nWorkFunction:%f\\nDetectorVoltage:%f\\nScreenVoltage:%f\\nConversionVoltage:%f\\nFocusDisplacement1:%f\\nFocusDisplacement2:%f\\nExposure:%u\\nGain:%u\\nBinning:%u\\nROIbottom:%u\\nROItop:%u\\nROIright:%u\\nROIleft:%u\\nDarkImg:%u\\nStartTime:%<%Y.%m.%d %H:%M:%S>T", initial string=w251, "delay" ("input 1"), w275, w276, w277, w255, w256, w257, w258, w259, w260, w261, w262, w263, w264, w265, w266, w267, w268, w269, w270, w271, w272, w273, w249) -> ()  [unwired: 1 in, 2 out]
          n230 = Less Or Equal?(x=w247, y=w248) -> (x <= y?=w279:bool)
          n231 = Or(x=w280, y=w279) -> (x .or. y?=w278:bool)
        }
        n232 = Build Path(base path=w231, name or relative path="scanvector.txt") -> (appended path=w228:path)
        n233 = call-poly <vilib>:"Write Delimited Spreadsheet.vi"("file path (dialog if empty)"=w228, "format (%.3f)"="%.6f", "1D data"=w224, "transpose? (no:F)"=TRUE ("transpose? (F)")) -> ()  [unwired: 10 in, 2 out]
        n234 = flat-sequence {
          tunnel: w227 -> [w421]
          tunnel: [w421] -> w226
          frame #0 {
            w420 = u32 1000 ("frequency (Hz)")
            n235 = call <vilib>:"Beep.vi"("use system alert? (T)"=FALSE, "duration (msec)"=w420, "frequency (Hz)"=w420) -> ()  [unwired: 9 in]
          }
        }
      }
      frame "refresh" {
        n236 = Dequeue Element(queue=w430) -> ()  [unwired: 2 in, 4 out]
        n237 = property on="mainimg" class="IntGraph (strict)"() -> ("CrsrLis"=w429:T5)  [unwired: 2 in, 2 out]
        n238 = Index Array(array=w428, index (dim 0)=0 ("disabled index (col)")) -> (element=w425:dbl[][][])  [unwired: 3 in]
        n239 = call "processData.vi"("Cursor List"=w429, "data in"=w425) -> ("Intensity Chart"=w427:dbl[])  [unwired: 1 in, 2 out]
        n240 = Bundle("delay pointss [fs]"=w426, "Intensity Chart"=w427) -> (w424:T6)  [unwired: 1 in]
        n241 = Build Array(w424) -> (w423:T3)
        n242 = local write "scangraph"(w423) -> ()
      }
      frame "manip" {
        n243 = Dequeue Element(queue=w461) -> (queue out=w460:refnum<queue>)  [unwired: 2 in, 3 out]
        n244 = local read "RunNumber"() -> (w469:u16)
        n245 = local read "BasePath"() -> (w470:path)
        n246 = property on="delscan_progress 2" class="Slide (strict)"("Scale.Maximum"="manip_scan_steps") -> ()  [unwired: 2 in, 2 out]
        n247 = Index Array(array="manip_scan_delta") -> (element #1=w482:dbl, element #2=w481:dbl, element #3=w480:dbl, element #4=w479:dbl, element #5=w478:dbl, element #6=w477:dbl)  [unwired: 6 in]
        n248 = Increment(x=w469) -> (x+1=w471:u16)
        n249 = Current VI's Path() -> (path=w468:path)
        n250 = Format Into String(format string="%g_%g_%g_%g_%g_%g", w482, w481, w480, w479, w478, w477) -> (resulting string=w475:string)  [unwired: 2 in, 1 out]
        n251 = property on="Mode" class="Enum (strict)"() -> ("RingText.Text"=w455:string)  [unwired: 2 in, 2 out]
        n252 = property on="VoltageRange" class="Enum (strict)"() -> ("RingText.Text"=w454:string)  [unwired: 2 in, 2 out]
        n253 = call "saverunnumber.vi"("RunNumber"=w471, "VI path"=w468) -> ()  [unwired: 10 in]
        n254 = local write "RunNumber"(w471) -> ()
        n255 = call "create_opti_path.vi"("RunNumber"=w471, "base path"=w470) -> ("Path"=w434:path)  [unwired: 2 in]
        n256 = local read "exposure [ms]"() -> (w444:u32)
        n257 = Build Path(base path=w434, name or relative path="info.txt") -> (appended path=w433:path)
        n258 = Concatenate Strings("relative:" ("string"), w475, ":wait" ("string")) -> (w484:string)
        n259 = local read "ROI Bottom"() -> (w441:i32)
        n260 = local read "cam_dark?"() -> (w458:bool)
        n261 = local read "phoib_I_1"() -> (w453:dbl)
        n262 = local read "phoib_I_2"() -> (w452:dbl)
        n263 = local read "phoib_I_3"() -> (w451:dbl)
        n264 = local read "phoib_I_4"() -> (w450:dbl)
        n265 = local read "phoib_I_5"() -> (w449:dbl)
        n266 = local read "phoib_I_6"() -> (w448:dbl)
        n267 = local read "phoib_I_7"() -> (w447:dbl)
        n268 = local read "phoib_I_8"() -> (w446:dbl)
        n269 = local read "phoib_I_9"() -> (w445:dbl)
        n270 = local read "ROI Right"() -> (w439:i32)
        n271 = local read "averages"() -> (w456:i32)
        n272 = local read "ROI Top"() -> (w440:i32)
        n273 = local read "ROI Left"() -> (w438:i32)
        n274 = local read "binning"() -> (w442:u16)
        n275 = local read "gain"() -> (w459:bool)
        n276 = Get Date/Time In Seconds() -> (seconds since 1Jan1904=w436:timestamp)
        n277 = Build Path(base path=w434, name or relative path="scanvector.txt") -> (appended path=w485:path)
        n278 = for {
          N: 1 -> [_]
          tunnel: w467 -> [w500]
          tunnel: w434 -> [w499]
          tunnel: w485 -> [w492]
          tunnel: "manip_scan_steps" -> [w491]
          tunnel: w484 -> [w490]
          tunnel: w465 -> [w489]
          tunnel: w460 -> [w488]
          tunnel: w466 -> [w487]
          tunnel: "manip_scan_delta" -> [w486]
          i -> [w494]
          n279 = Add(x=w494, y=1000) -> (x+y=w497:i32)
          n280 = Number To Decimal String(number=w497) -> (decimal integer string=w496:string)  [unwired: 1 in]
          n281 = String Subset(string=w496, offset (0)=1) -> (substring=w493:string)  [unwired: 1 in]
          n282 = for {
            N: w491 -> [_]
            tunnel: w500 -> [w525]
            tunnel: w499 -> [w522]
            tunnel: w493 -> [w516]
            tunnel: w492 -> [w518]
            tunnel: w490 -> [w513]
            tunnel: w489 -> [w512]
            tunnel: w488 -> [w511]
            tunnel: w487 -> [w510]
            tunnel: w486 -> [w508]
            i -> [w503]
            stop <- "abort" stop-if-true
            n283 = Increment(x=w503) -> (x+1=→"delscan_progress 2":i32)
            n284 = Multiply(x=w508, y=w503) -> (x*y=w507:dbl[])
            n285 = Enqueue Element(queue=w512, element=w513) -> (error out=w514:errorcluster)  [unwired: 2 in, 2 out]
            n286 = Add(x=w503, y=10000) -> (x+y=w531:i32)
            n287 = Dequeue Element(queue=w511, error in (no error)=w514) -> (error out=w509:errorcluster)  [unwired: 1 in, 3 out]
            n288 = Number To Decimal String(number=w531) -> (decimal integer string=w530:string)  [unwired: 1 in]
            n289 = String Subset(string=w530, offset (0)=1) -> (substring=w515:string)  [unwired: 1 in]
            n290 = Enqueue Element(queue=w510, element="snap", error in (no error)=w509) -> (error out=w524:errorcluster)  [unwired: 1 in, 2 out]
            n291 = Concatenate Strings("RAW\\" ("string"), w516, "_" ("string"), w515, ".tsv" ("string")) -> (w521:string)
            n292 = Dequeue Element(queue=w525, error in (no error)=w524) -> (element=w520:dbl[][][])  [unwired: 1 in, 3 out]
            n293 = Build Path(base path=w522, name or relative path=w521) -> (appended path=w523:path)
            n294 = Index Array(array=w520, index (dim 2)=0 ("disabled index (col)")) -> (element=w502:dbl[][])  [unwired: 2 in]
            n295 = call-poly <vilib>:"Write Delimited Spreadsheet.vi"("file path (dialog if empty)"=w523, "2D data"=w502) -> ()  [unwired: 12 in, 2 out]
            n296 = call-poly <vilib>:"Write Delimited Spreadsheet.vi"("file path (dialog if empty)"=w518, "1D data"=w507, "append to file? (new file:F)"=TRUE ("append to file? (F)"), "transpose? (no:F)"=FALSE ("transpose? (F)")) -> ()  [unwired: 10 in, 2 out]
          }
        }
        n297 = Boolean To (0,1)(Boolean=w459) -> (0, 1=w443:i16)
        n298 = Boolean To (0,1)(Boolean=w458) -> (0, 1=w437:i16)
        n299 = Format Into String(format string="ScanType:%s\\nAverages:%u\\nMode:%s\\nVoltageRange:%s\\nKineticEnergy:%f\\nPassEnergy:%f\\nCoilCurrent:%f\\nWorkFunction:%f\\nDetectorVoltage:%f\\nScreenVoltage:%f\\nConversionVoltage:%f\\nFocusDisplacement1:%f\\nFocusDisplacement2:%f\\nExposure:%u\\nGain:%u\\nBinning:%u\\nROIbottom:%u\\nROItop:%u\\nROIright:%u\\nROIleft:%u\\nDarkImg:%u\\nStartTime:%<%Y.%m.%d %H:%M:%S>T", initial string=w433, "manipulator" ("input 1"), w456, w455, w454, w453, w452, w451, w450, w449, w448, w447, w446, w445, w444, w443, w442, w441, w440, w439, w438, w437, w436) -> ()  [unwired: 1 in, 2 out]
      }
      frame "single" {
        n300 = Dequeue Element(queue=w577) -> ()  [unwired: 2 in, 4 out]
        n301 = property on="Mode" class="Enum (strict)"() -> ("RingText.Text"=w562:string)  [unwired: 2 in, 2 out]
        n302 = property on="VoltageRange" class="Enum (strict)"() -> ("RingText.Text"=w561:string)  [unwired: 2 in, 2 out]
        n303 = local read "RunNumber"() -> (w568:u16)
        n304 = local read "BasePath"() -> (w569:path)
        n305 = local read "exposure [ms]"() -> (w551:u32)
        n306 = local read "ROI Bottom"() -> (w548:i32)
        n307 = local read "cam_dark?"() -> (w565:bool)
        n308 = local read "phoib_I_1"() -> (w560:dbl)
        n309 = local read "phoib_I_2"() -> (w559:dbl)
        n310 = local read "phoib_I_3"() -> (w558:dbl)
        n311 = local read "phoib_I_4"() -> (w557:dbl)
        n312 = local read "phoib_I_5"() -> (w556:dbl)
        n313 = local read "phoib_I_6"() -> (w555:dbl)
        n314 = local read "phoib_I_7"() -> (w554:dbl)
        n315 = local read "phoib_I_8"() -> (w553:dbl)
        n316 = local read "phoib_I_9"() -> (w552:dbl)
        n317 = local read "ROI Right"() -> (w546:i32)
        n318 = local read "ESP_pos"() -> (w535:dbl)
        n319 = local read "averages"() -> (w563:i32)
        n320 = local read "ROI Top"() -> (w547:i32)
        n321 = local read "ROI Left"() -> (w545:i32)
        n322 = local read "binning"() -> (w549:u16)
        n323 = local read "ESP_t0"() -> (w536:dbl)
        n324 = Increment(x=w568) -> (x+1=w570:u16)
        n325 = Current VI's Path() -> (path=w567:path)
        n326 = local read "gain"() -> (w566:bool)
        n327 = Get Date/Time In Seconds() -> (seconds since 1Jan1904=w543:timestamp)
        n328 = call "saverunnumber.vi"("RunNumber"=w570, "VI path"=w567) -> ()  [unwired: 10 in]
        n329 = local write "RunNumber"(w570) -> ()
        n330 = call "create_opti_path.vi"("RunNumber"=w570, "base path"=w569) -> ("Path"=w540:path)  [unwired: 2 in]
        n331 = Boolean To (0,1)(Boolean=w566) -> (0, 1=w550:i16)
        n332 = Boolean To (0,1)(Boolean=w565) -> (0, 1=w544:i16)
        n333 = Build Path(base path=w540, name or relative path="info.txt") -> (appended path=w538:path)
        n334 = Format Into String(format string="ScanType=%s\\nDelayPosition=%.6f\\nTimeZero=%.6f\\nAverages=%u\\nLensMode=%s\\nVoltageRange=%s\\nKineticEnergy=%f\\nPassEnergy=%f\\nCoilCurrent=%f\\nWorkFunction=%f\\nDetectorVoltage=%f\\nScreenVoltage=%f\\nConversionVoltage=%f\\nFocusDisplacement1=%f\\nFocusDisplacement2=%f\\nExposure=%u\\nGain=%u\\nBinning=%u\\nROIbottom=%u\\nROItop=%u\\nROIright=%u\\nROIleft=%u\\nDarkImg=%u\\nStartTime=%<%Y.%m.%d %H:%M:%S>T", initial string=w538, "single" ("input 1"), w535, w536, w563, w562, w561, w560, w559, w558, w557, w556, w555, w554, w553, w552, w551, w550, w549, w548, w547, w546, w545, w544, w543) -> ()  [unwired: 1 in, 2 out]
        n335 = Build Path(base path=w540, name or relative path="AVG\\000.tsv") -> (appended path=w541:path)
        n336 = Enqueue Element(queue=w578, element="snap" ("string")) -> (error out=w572:errorcluster)  [unwired: 2 in, 2 out]
        n337 = Dequeue Element(queue=w576, error in (no error)=w572) -> (element=w571:dbl[][][])  [unwired: 1 in, 3 out]
        n338 = Index Array(array=w571, index (dim 2)=0 ("disabled index (col)")) -> (element=w534:dbl[][])  [unwired: 2 in]
        n339 = call-poly <vilib>:"Write Delimited Spreadsheet.vi"("file path (dialog if empty)"=w541, "2D data"=w534) -> ()  [unwired: 12 in, 2 out]
      }
    }
  }
  n340 = while {
    tunnel: w10 -> [w605]
    shift-right: [w599] -> _
    shift-left: _ -> [w598]
    shift-right: [w597] -> _
    shift-left: _ -> [w595]
    shift-right: [w596] -> _
    shift-left: _ -> [w594]
    shift-right: [w591] -> _
    shift-left: 0 -> [w592]
    shift-right: [w590] -> _
    shift-left: _ -> [w589]
    shift-right: [w588] -> _
    shift-left: _ -> [w587]
    tunnel: w11 -> [w586]
    shift-right: [w585] -> _
    shift-left: _ -> [w584]
    shift-right: [w582] -> _
    shift-left: _ -> [w581]
    shift-right: [w580] -> _
    shift-left: _ -> [w579]
    i -> [w583]
    stop <- w593 stop-if-true
    # "cam"
    n341 = Preview Queue Element(queue=w605, timeout in ms (-1)=w592) -> (queue out=w604:refnum<queue>, element=w603:string)  [unwired: 1 in, 2 out]
    n342 = Match Pattern(string=w603, regular expression=":") -> (before substring=w600:string, after substring=w601:string)  [unwired: 1 in, 2 out]
    n343 = case shown="\"close\"" w600 {
      tunnel: w604 -> [w618 w650 w680 w720 w733 _ w821 w854 w964]
      tunnel: w601 -> [_ _ _ _ _ _ _ _ _]
      tunnel: [w612 w637 w676 w719 w731 w774 w818 w839 w962] -> w599
      tunnel: w598 -> [_ _ w676 w719 w731 w774 w818 w839 w962]
      tunnel: [w617 w651 w686 u64 0 ("Hout") w730 w778 w819 w849 w961] -> w597
      tunnel: [w619 w652 w687 w716 w729 w779 w820 w840 w960] -> w596
      tunnel: w595 -> [_ w654 w690 w718 w730 w781 w823 w851 w961]
      tunnel: w594 -> [_ w653 w682 _ w729 w780 w822 w850 w960]
      tunnel: [_ _ _ _ TRUE _ _ _ _] -> w593
      tunnel: [_ _ _ _ _ _ _ _ -1] -> w591
      tunnel: [w611 w638 w681 _ _ w788 _ _ _] -> w590
      tunnel: w589 -> [w611 w638 w681 _ _ w787 _ _ _]
      tunnel: [w612 w640 w683 w714 w728 w783 w812 w852 w959] -> w588
      tunnel: w587 -> [_ w640 w683 w714 w728 w783 _ w852 w959]
      tunnel: w586 -> [_ _ _ _ _ _ _ w843 _]
      tunnel: [w609 w635 w685 w713 w726 w741 w809 w846 w958] -> w585
      tunnel: w584 -> [w609 w635 w685 w713 w726 w776 w809 w846 w958]
      tunnel: w583 -> [_ _ _ _ _ w749 _ _ _]
      tunnel: [w610 w636 w684 w712 w727 w775 w808 w845 w957] -> w582
      tunnel: w581 -> [w610 w636 w684 w712 w727 w748 w808 w845 w957]
      tunnel: [w606 w632 w670 refnum<k21> refnum ("task out") w725 w734 w807 w836 w956] -> w580
      tunnel: w579 -> [_ w632 w671 w711 w725 w734 w807 w837 w956]
      frame "init" {
        w607 = 10106 items=["Default"=-1, "RSE"=10083, "NRSE"=10078, "Differential"=10106, "Pseudodifferential"=12529] ("input terminal configuration")
        w612 = u16[][] []
        n344 = flat-sequence {
          tunnel: [w621] -> w616
          tunnel: [w622] -> w615
          tunnel: [w630] -> w617
          tunnel: [w631] -> w619
          tunnel: w616 -> [w631]
          tunnel: w615 -> [w630]
          frame #0 {
            n345 = local write "cam_con?"(FALSE ("cam_con?")) -> ()
          }
          frame #1 {
            n346 = call "SCInitBoard.vi"("boardnr"="board number") -> ("Hout"=w625:u32, "error out"=w626:errorcluster)  [unwired: 1 in, 1 out]
            n347 = call "SCSetupCamera.vi"("Handle"=w625, "error in (no error)"=w626) -> ("Hout"=w627:u64, "error out"=w628:errorcluster)  [unwired: 1 out]
            n348 = call "SCStopCOC.vi"("error in (no error)"=w628, "Stop mode"=0, "Handle"=w627) -> ("error out"=w621:errorcluster, "Hout"=w622:u64)
          }
          frame #2 {
            n349 = local write "cam_con?"(TRUE ("cam_con?")) -> ()
          }
        }
        n350 = Dequeue Element(queue=w618) -> (queue out=w614:refnum<queue>)  [unwired: 2 in, 3 out]
        n351 = Enqueue Element At Opposite End(queue=w614, element="set") -> ()  [unwired: 2 in, 3 out]
        n352 = call-poly <vilib>:"DAQmx Create Virtual Channel.vi"("input terminal configuration"=w607, "physical channels"=tag "Dev2/ai0") -> ("task out"=w606:refnum<k21>)  [unwired: 12 in, 1 out]
      }
      frame "set" {
        n353 = Dequeue Element(queue=w650) -> ()  [unwired: 2 in, 4 out]
        n354 = call "SCStopCOC.vi"("error in (no error)"=w653, "Stop mode"=0, "Handle"=w654) -> ("error out"=w669:errorcluster, "Hout"=w668:u64)
        n355 = Bundle By Name(cluster=cluster{"Delay":dbl, "Exposure ":dbl} {"Delay"=0.0, "Exposure "=0.0} ("Delay and exposure"), "Exposure"="exposure [ms]") -> (w647:cluster{"Delay":dbl, "Exposure ":dbl})
        n356 = Bundle By Name(cluster=T7 {"Camera type"=0, "Operating mode\nHP & QE / HS & DiCam Pro "=0, "Frame trigger \n(High Performance and QE only)"=0, "Sequence trigger"=0, "Low Light\n(QE only)"=FALSE, "Gain"=FALSE, "Horzontal\nbinning"=0, "Vertical\nbinning "=0, "ROI Left"=1, "ROI Right"=20, "ROI Top"=1, "ROI Bottom"=15} ("Camera controls"), "Operating mode\nHP & QE / HS & DiCam Pro"="Operating mode\nHP & QE / HS & DiCam Pro", "Horzontal\nbinning"="binning", "Vertical\nbinning"="binning", "ROI Left"="ROI Left", "ROI Right"="ROI Right", "ROI Top"="ROI Top", "ROI Bottom"="ROI Bottom", "Gain"="gain", "Frame trigger \n(High Performance and QE only)"="Frame trigger \n(High Performance and QE only)") -> (w664:T7)
        n357 = call "New delay and exposure forma.vi"("Operating mode\nHP & QE / HS & DiCam Pro"="Operating mode\nHP & QE / HS & DiCam Pro", "Delay and exposure"=w647) -> ("Output table"=w665:string)  [unwired: 3 in]
        n358 = call "SCSetCoC.vi"("error in (no error)"=w669, "Delay and exposure table"=w665, "Camera controls"=w664, "Handle"=w668) -> ("error out"=w657:errorcluster, "Hout"=w656:u64)  [unwired: 1 out]
        n359 = call "SCGetImageSize.vi"("Handle"=w656, "error in (no error)"=w657) -> ("Hout"=w655:u64, "error out"=w639:errorcluster, "Horizontal size"=w644:i32, "Vertical size"=w643:i32)  [unwired: 2 out]
        n360 = Greater?(x=w644, y=w643) -> (0:w645:bool)
        n361 = Initialize Array(u16 0 ("dimension size"), w643, w644) -> (w637:u16[][])
        n362 = call "SCRun.vi"("error in (no error)"=w639, "Run mode"=0, "Handle"=w655) -> ("error out"=w652:errorcluster, "Hout"=w651:u64)  [unwired: 1 out]
        n363 = Select(t=w644, s=w645, f=w643) -> (s? t:f=w642:i32)
        n364 = property on="mainimg" class="IntGraph (strict)"("XScale.Maximum"=w642, "YScale.Maximum"=w642) -> ()  [unwired: 2 in, 2 out]
      }
      frame "bench" {
        n365 = Dequeue Element(queue=w680) -> ()  [unwired: 2 in, 4 out]
        n366 = call "SCStopCOC.vi"("error in (no error)"=w682, "Stop mode"=0, "Handle"=w690) -> ("error out"=w674:errorcluster, "Hout"=w675:u64)
        n367 = while {
          tunnel: w676 -> [w706]
          tunnel: w675 -> [w705]
          tunnel: w674 -> [w696]
          shift-right: [w702] -> _
          shift-left: _ -> [w701]
          tunnel: [w698] -> w673
          tunnel: [w697] -> w672
          tunnel: w671 -> [w693]
          tunnel: [w692] -> w670
          stop <- "stop" stop-if-true
          n368 = call "wait4trig.vi"("error in"=w696, "task/channels in"=w693) -> ("error out"=w695:errorcluster, "voltage out"=→"voltage out":dbl, "task out"=w692:refnum<k21>)  [unwired: 7 in]
          n369 = call "SCRun.vi"("error in (no error)"=w695, "Run mode"=4, "Handle"=w705) -> ("error out"=w707:errorcluster, "Hout"=w708:u64)  [unwired: 1 out]
          n370 = call <vilib>:"High Resolution Relative Seconds.vi"() -> ("relative seconds"=w702:dbl)
          n371 = call "grabimg.vi"("array in"=w706, "error in"=w707, "Hin"=w708) -> ("error out"=w697:errorcluster, "imgdata"=w704:i32[][], "Hout"=w698:u64)  [unwired: 6 in]
          n372 = To Double Precision Float(number=w704) -> (double precision float=→"sideimg 2":dbl[][])
          n373 = Subtract(x=w702, y=w701) -> (x-y=w699:dbl)
          "x/y" <- w699
          n374 = Reciprocal(x=w699) -> (1/x=→"1/x":dbl)
        }
        n375 = call "SCStopCOC.vi"("error in (no error)"=w672, "Stop mode"=0, "Handle"=w673) -> ("error out"=w677:errorcluster, "Hout"=w678:u64)
        n376 = call "SCRun.vi"("error in (no error)"=w677, "Run mode"=0, "Handle"=w678) -> ("error out"=w687:errorcluster, "Hout"=w686:u64)  [unwired: 1 out]
      }
      frame "release" {
        n377 = Dequeue Element(queue=w720) -> ()  [unwired: 2 in, 4 out]
        n378 = flat-sequence {
          tunnel: w718 -> [w722]
          tunnel: [w721] -> w715
          tunnel: [w724] -> w716
          tunnel: w715 -> [w724]
          frame #0 {
            n379 = call "SCCloseBoard.vi"("Handle"=w722) -> ("error out"=w721:errorcluster)  [unwired: 1 in, 2 out]
          }
          frame #1 {
            n380 = local write "cam_con?"(FALSE ("cam_con?")) -> ()
          }
        }
        n381 = call <vilib>:"DAQmx Clear Task.vi"("task in"=w711) -> ()  [unwired: 14 in, 1 out]
      }
      frame "close" {
        n382 = Release Queue(queue=w733) -> ()  [unwired: 2 in, 3 out]
      }
      frame "idle", Default {
        n383 = call "grabimg.vi"("array in"=w774, "error in"=w780, "Hin"=w781) -> ("error out"=w779:errorcluster, "imgdata"=w777:i32[][], "Hout"=w778:u64)  [unwired: 6 in]
        n384 = local read "lower threshold"() -> (w772:i32)
        n385 = case shown="False" "cam_dark?" {
          tunnel: w783 -> [_ w806]
          tunnel: [w803 w805] -> w773
          tunnel: w777 -> [w803 w804]
          frame False {
          }
          frame True {
            n386 = Subtract(x=w804, y=w806) -> (x-y=w805:dbl[][])
          }
        }
        n387 = call "filtr_b.vi"("threshold"=w772, "input array"=w773) -> ("output array"=w764:dbl[][])  [unwired: 9 in]
        n388 = call <vilib>:"High Resolution Relative Seconds.vi"() -> ("relative seconds"=w788:dbl)
        n389 = Subtract(x=w788, y=w787) -> (x-y=w786:dbl)
        n390 = Array Size(array=w764) -> (size(s)=w763:i32[])
        n391 = Reciprocal(x=w786) -> (1/x=→"cam_fps":dbl)
        n392 = Index Array(array=w763) -> (element #1=w758:i32, element #2=w757:i32)  [unwired: 2 in]
        n393 = Subtract(x=w749, y=w748) -> (x-y=w747:i32)
        n394 = Less Or Equal?(x="pics2avg", y=w747) -> (x <= y?=w770:bool)
        n395 = And(x="reset every n pics", y=w770) -> (x .and. y?=w768:bool)
        n396 = Not(x=w768) -> (.not. x?=w767:bool)
        n397 = call-poly <vilib>:"Ramp Pattern.vi"("start"=0.0, "end"=w758, "samples"=w758) -> ("Ramp Pattern"=w753:dbl[])  [unwired: 7 in, 1 out]
        n398 = call-poly <vilib>:"Ramp Pattern.vi"("start"=0.0, "end"=w757, "samples"=w757) -> ("Ramp Pattern"=w754:dbl[])  [unwired: 7 in, 1 out]
        n399 = property on="mainimg" class="IntGraph (strict)"() -> ("CrsrLis"=w746:T5)  [unwired: 2 in, 2 out]
        n400 = And(x="cam_liveavg", y=w767) -> (x .and. y?=w765:bool)
        n401 = case shown="False" w765 {
          tunnel: w764 -> [w793 w799]
          tunnel: [w793 w796] -> w741
          tunnel: w776 -> [_ w801]
          tunnel: w749 -> [w794 _]
          tunnel: [w794 w802] -> w775
          tunnel: w748 -> [_ w802]
          tunnel: w747 -> [_ w795]
          frame False {
          }
          frame True {
            n402 = Multiply(x=w801, y=w795) -> (x*y=w800:dbl[][])
            n403 = Increment(x=w795) -> (x+1=w797:i32)
            n404 = Add(x=w800, y=w799) -> (x+y=w798:dbl[][])
            n405 = Divide(x=w798, y=w797) -> (x/y=w796:dbl[][])
          }
        }
        "mainimg" <- w741
        n406 = Index Array(array=w746) -> (element #1=w744:T8, element #2=w745:T8)  [unwired: 2 in]
        n407 = Unbundle By Name(w744) -> ("Position.X"=w738:dbl, "Position.Y"=w740:dbl)
        n408 = Unbundle By Name(w745) -> ("Position.X"=w742:dbl, "Position.Y"=w743:dbl)
        n409 = Array Max & Min(array=w741) -> (max value=→"max":dbl)  [unwired: 3 out]
        n410 = Subtract(x=w743, y=w740) -> (x-y=w739:dbl)
        n411 = Subtract(x=w742, y=w738) -> (x-y=w737:dbl)
        n412 = Array Subset(array=w741, index (row)=w740, length (row)=w739) -> (w752:dbl[][])  [unwired: 2 in]
        n413 = Array Subset(array=w741, index (col)=w738, length (col)=w737) -> (w750:dbl[][])  [unwired: 2 in]
        n414 = Array Subset(array=w741, index (row)=w740, length (row)=w739, index (col)=w738, length (col)=w737) -> (w736:dbl[][])
        n415 = Transpose 2D Array(2D array=w752) -> (transposed array=w751:dbl[][])
        n416 = Add Array Elements(numeric array=w736) -> (sum=→"sum" →"Waveform Chart":dbl)
        n417 = for {
          tunnel: w750 -> [w790] mode=indexing
          tunnel: [w789] -> w760 mode=indexing
          n418 = Add Array Elements(numeric array=w790) -> (sum=w789:dbl)
        }
        n419 = for {
          tunnel: w751 -> [w792] mode=indexing
          tunnel: [w791] -> w759 mode=indexing
          n420 = Add Array Elements(numeric array=w792) -> (sum=w791:dbl)
        }
        n421 = Bundle("Ramp Pattern"=w754, w759) -> (→"G2 X":cluster{"Ramp Pattern":dbl[], dbl[]})  [unwired: 1 in]
        n422 = Bundle(w760, "Ramp Pattern"=w753) -> (→"G2 Y":cluster{dbl[], "Ramp Pattern":dbl[]})  [unwired: 1 in]
      }
      frame "dark" {
        n423 = Dequeue Element(queue=w821) -> ()  [unwired: 2 in, 4 out]
        n424 = Array Size(array=w818) -> (size(s)=w817:i32[])
        n425 = Index Array(array=w817) -> (element #1=w816:i32, element #2=w815:i32)  [unwired: 2 in]
        n426 = Initialize Array(0.0 ("element"), w816, w815) -> (w813:dbl[][])
        n427 = for {
          N: "dark avg" -> [_]
          tunnel: w823 -> [w831]
          tunnel: w822 -> [w830]
          tunnel: [w829] -> w820
          tunnel: w818 -> [w828]
          tunnel: [w827] -> w819
          shift-right: [w824] -> w811
          shift-left: w813 -> [w825]
          n428 = call "grabimg.vi"("array in"=w828, "error in"=w830, "Hin"=w831) -> ("error out"=w829:errorcluster, "imgdata"=w826:i32[][], "Hout"=w827:u64)  [unwired: 6 in]
          n429 = Add(x=w826, y=w825) -> (x+y=w824:dbl[][])
        }
        n430 = Divide(x=w811, y="dark avg") -> (x/y=w812:dbl[][])
      }
      frame "snap" {
        w835 = 0
        n431 = Dequeue Element(queue=w854) -> ()  [unwired: 2 in, 4 out]
        n432 = local read "cam_dark?"() -> (w853:bool)
        n433 = local read "averages"() -> (w848:i32)
        n434 = To Double Precision Float(number=w839) -> (double precision float=w838:dbl[][])
        n435 = Equal To 0?(x="aq.mode") -> (x = 0?=w841:bool)
        n436 = Get Date/Time In Seconds() -> (seconds since 1Jan1904=w844:timestamp)
        n437 = for {
          N: w848 -> [w874]
          shift-right: [w892] -> w849
          shift-left: w851 -> [w894]
          shift-right: [w879] -> w847
          shift-left: w850 -> [w893]
          tunnel: w853 -> [w890]
          tunnel: w852 -> [w889]
          tunnel: w839 -> [w888]
          tunnel: w844 -> [w884]
          tunnel: w841 -> [w867]
          shift-right: [w875] -> w832
          shift-left: w838 -> [w876]
          shift-right: [w860] -> w834
          shift-left: w838 -> [w866]
          shift-right: [w865] -> w836
          shift-left: w837 -> [w859]
          shift-right: [w856] -> _
          shift-left: w835 -> [w857]
          shift-right: [w855] -> _
          shift-left: w835 -> [w858]
          i -> [w863]
          stop <- "abort acq." stop-if-true
          n438 = call "grabimg.vi"("array in"=w888, "error in"=w893, "Hin"=w894) -> ("error out"=w879:errorcluster, "imgdata"=w891:i32[][], "Hout"=w892:u64)  [unwired: 6 in]
          n439 = local read "lower threshold"() -> (w870:i32)
          n440 = Increment(x=w863) -> (x+1=w872:i32)
          "acq. imgs" <- w872
          n441 = Get Date/Time In Seconds() -> (seconds since 1Jan1904=w887:timestamp)
          n442 = case shown="True" w890 {
            tunnel: w891 -> [w952 w955]
            tunnel: w889 -> [_ w954]
            tunnel: [w952 w953] -> w869
            frame False {
            }
            frame True {
              n443 = Subtract(x=w955, y=w954) -> (x-y=w953:dbl[][])
            }
          }
          n444 = Divide(x=w872, y=w874) -> (x/y=→"snap_prog":dbl)
          n445 = flat-sequence {
            tunnel: [w895] -> w865
            tunnel: [w899] -> w864
            tunnel: w862 -> [w898]
            tunnel: [w898] -> w861
            tunnel: [w897] -> _
            tunnel: w859 -> [w897]
            frame #0 {
              n446 = call-poly <vilib>:"DAQmx Read.vi"("task/channels in"=w897) -> ("task out"=w895:refnum<k21>, "data"=w896:dbl)  [unwired: 12 in, 1 out]
              "Voltage" <- w896
              n447 = Greater?(x=w896, y=2.5) -> (0:w899:bool)
            }
          }
          n448 = Subtract(x=w887, y=w884) -> (x-y=w886:dbl)
          n449 = call "filtr_b.vi"("threshold"=w870, "input array"=w869) -> ("output array"=w868:dbl[][])  [unwired: 9 in]
          n450 = Divide(x=w886, y=w863) -> (x/y=w882:dbl)
          n451 = Multiply(x=w882, y=w874) -> (x*y=w885:dbl)
          n452 = Reciprocal(x=w882) -> (1/x=w881:dbl)
          n453 = case shown="True" "count?" {
            tunnel: w868 -> [w941 w943]
            tunnel: "e-size" -> [_ w945]
            tunnel: w870 -> [_ w944]
            tunnel: [w941 w942] -> w862
            frame False {
            }
            frame True {
              n454 = Array Size(array=w943) -> (size(s)=w947:i32[])
              n455 = call "findr.vi"("thresh"=w944, "esize"=w945, "inp array"=w943) -> ("locs"=w946:i32[][])  [unwired: 8 in]
              n456 = Index Array(array=w947) -> (element #1=w949:i32, element #2=w948:i32)  [unwired: 2 in]
              n457 = call "drawe.vi"("Ysize"=w949, "Xsize"=w948, "pos array"=w946) -> ("img out"=w942:i32[][])  [unwired: 8 in]
            }
          }
          n458 = Add(x=w885, y=w884) -> (x+y=→"ETA":timestamp)
          n459 = local write "cam_fps"(w881) -> ()
          n460 = case shown="False" w864 {
            tunnel: w867 -> [w906 _]
            tunnel: w866 -> [w905 w920]
            tunnel: [w904 w920] -> w860
            tunnel: w861 -> [w903 _]
            tunnel: w858 -> [w902 w919]
            tunnel: [w901 w919] -> w855
            frame False {
              n461 = case shown="False" w906 {
                tunnel: w903 -> [w909 w917]
                tunnel: w902 -> [w908 w916]
                tunnel: w905 -> [w911 w915]
                tunnel: [w910 w913] -> w904
                tunnel: [w907 w912] -> w901
                frame False {
                  n462 = Add(x=w909, y=w911) -> (x+y=w910:dbl[][])
                  n463 = Increment(x=w908) -> (x+1=w907:i32)
                }
                frame True {
                  n464 = Multiply(x=w915, y=w916) -> (x*y=w918:dbl[][])
                  n465 = Increment(x=w916) -> (x+1=w912:i32)
                  n466 = Add(x=w917, y=w918) -> (x+y=w914:dbl[][])
                  n467 = Divide(x=w914, y=w912) -> (x/y=w913:dbl[][])
                }
              }
            }
            frame True {
            }
          }
          "Pics NL" <- w855
          n468 = case shown="True" w864 {
            tunnel: w876 -> [w922 w928]
            tunnel: [w922 w927] -> w875
            tunnel: w867 -> [_ w926]
            tunnel: w861 -> [_ w925]
            tunnel: w857 -> [w921 w924]
            tunnel: [w921 w923] -> w856
            frame False {
            }
            frame True {
              n469 = case shown="True" w926 {
                tunnel: w925 -> [w931 w939]
                tunnel: w924 -> [w930 w938]
                tunnel: w928 -> [w933 w937]
                tunnel: [w932 w935] -> w927
                tunnel: [w929 w934] -> w923
                frame False {
                  n470 = Add(x=w931, y=w933) -> (x+y=w932:dbl[][])
                  n471 = Increment(x=w930) -> (x+1=w929:i32)
                }
                frame True {
                  n472 = Multiply(x=w937, y=w938) -> (x*y=w940:dbl[][])
                  n473 = Increment(x=w938) -> (x+1=w934:i32)
                  n474 = Add(x=w939, y=w940) -> (x+y=w936:dbl[][])
                  n475 = Divide(x=w936, y=w934) -> (x/y=w935:dbl[][])
                }
              }
            }
          }
          "Pics L" <- w856
          n476 = local write "mainimg"(w868) -> ()
          n477 = Transpose 2D Array(2D array=w868) -> (transposed array=w880:dbl[][])
          n478 = for {
            tunnel: w880 -> [w951] mode=indexing
            tunnel: [w950] -> _ mode=indexing
            n479 = Add Array Elements(numeric array=w951) -> (sum=w950:dbl)
          }
          n480 = local write "sideimg"(w875) -> ()
          n481 = local write "sideimg 2"(w860) -> ()
        }
        n482 = Build Array(w832, w834) -> (w833:dbl[][][])
        n483 = Enqueue Element(queue=w843, element=w833, error in (no error)=w847) -> (error out=w840:errorcluster)  [unwired: 1 in, 2 out]
      }
      frame "suspend" {
        n484 = Dequeue Element(queue=w964) -> ()  [unwired: 2 in, 4 out]
      }
    }
    "cam_error" <- w596
  }
  n485 = while {
    tunnel: w10 -> [w970]
    tunnel: w13 -> [w969]
    tunnel: w3 -> [w968]
    tunnel: w24 -> [w967]
    tunnel: w2 -> [w965]
    tunnel: w11 -> [w966]
    stop <- w971 stop-if-true
    n486 = event shown="[20] \"ESP_dest\": Value Change" {
      selector: _ -> [_ _ _ _ _ _ _ _ _ _ _ _ _ _ _ _ _ _ _ _ _ _ _ _ _ _ _]
      dyn-events: _ -> [_ _ _ _ _ _ _ _ _ _ _ _ _ _ _ _ _ _ _ _ _ _ _ _ _ _ _]
      timeout: _ -> [_ _ _ _ _ _ _ _ _ _ _ _ _ _ _ _ _ _ _ _ _ _ _ _ _ _ _]
      tunnel: [_ TRUE _ _ _ _ _ _ _ _ _ _ _ _ _ _ _ _ _ _ _ _ _ _ _ _ _] -> w971
      tunnel: w970 -> [_ w984 w987 _ _ _ _ _ w1013 w1015 _ _ _ _ _ _ _ _ _ _ _ _ _ _ _ _ w1122]
      tunnel: w969 -> [_ w983 _ w991 _ _ _ _ _ _ _ _ _ _ _ _ _ w1048 _ w1060 _ _ _ _ _ _ _]
      tunnel: w968 -> [_ w982 _ _ w997 _ _ _ _ _ _ _ _ _ w1036 _ w1040 _ _ _ _ _ _ _ _ _ _]
      tunnel: w967 -> [_ w981 _ _ _ w1003 w1009 w1010 _ _ _ _ _ _ _ _ _ _ _ _ _ _ _ _ _ _ _]
      tunnel: w966 -> [_ w975 _ _ _ _ _ _ _ _ _ _ _ _ _ _ _ _ _ _ _ _ _ _ _ _ _]
      tunnel: w965 -> [_ w974 _ _ _ _ _ _ _ _ w1017 w1019 w1020 _ _ w1038 _ _ _ _ _ _ _ _ _ w1121 _]
      event Timeout {
        n487 = event-data() -> ()  [unwired: 1 in, 1 out]
        n488 = call-poly <vilib>:"Read Delimited Spreadsheet.vi"() -> ("all rows"=w972:string[][])  [unwired: 10 in, 5 out]
        n489 = local write "delay table [fs]"(w972) -> ()
      }
      event "main_close": Value Change {
        w973 = "close" ("element")
        w980 = "release" ("element")
        n490 = event-data() -> ()  [unwired: 1 in, 1 out]
        n491 = Release Queue(queue=w975) -> ()  [unwired: 2 in, 3 out]
        n492 = Enqueue Element(queue=w984, element=w980) -> (queue out=w979:refnum<queue>)  [unwired: 2 in, 2 out]
        n493 = Enqueue Element(queue=w983, element=w980) -> (queue out=w978:refnum<queue>)  [unwired: 2 in, 2 out]
        n494 = Enqueue Element(queue=w982, element=w980) -> (queue out=w977:refnum<queue>)  [unwired: 2 in, 2 out]
        n495 = Enqueue Element(queue=w981, element=w980) -> (queue out=w976:refnum<queue>)  [unwired: 2 in, 2 out]
        n496 = Enqueue Element(queue=w979, element=w973) -> ()  [unwired: 2 in, 3 out]
        n497 = Enqueue Element(queue=w978, element=w973) -> ()  [unwired: 2 in, 3 out]
        n498 = Enqueue Element(queue=w977, element=w973) -> ()  [unwired: 2 in, 3 out]
        n499 = Enqueue Element(queue=w976, element=w973) -> ()  [unwired: 2 in, 3 out]
        n500 = Enqueue Element(queue=w974, element=w973) -> ()  [unwired: 2 in, 3 out]
      }
      event "cam_release", "cam_init": Value Change {
        n501 = event-data() -> ()  [unwired: 1 in, 2 out]
        n502 = Select(t="init" ("name (unnamed)"), s="cam_init", f="release" ("name (unnamed)")) -> (s? t:f=w986:string)
        n503 = Enqueue Element(queue=w987, element=w986) -> ()  [unwired: 2 in, 3 out]
      }
      event "ESP_release", "ESP_init": Value Change {
        n504 = event-data() -> ()  [unwired: 1 in, 2 out]
        n505 = Select(t="init" ("name (unnamed)"), s="ESP_init", f="release" ("name (unnamed)")) -> (s? t:f=w995:string)
        n506 = Enqueue Element(queue=w991, element=w995) -> ()  [unwired: 2 in, 3 out]
      }
      event "manip_init", "manip_release": Value Change {
        n507 = event-data() -> ()  [unwired: 1 in, 2 out]
        n508 = Flush Queue(queue=w997) -> (queue out=w996:refnum<queue>)  [unwired: 1 in, 2 out]
        n509 = Select(t="init" ("name (unnamed)"), s="manip_init", f="release" ("name (unnamed)")) -> (s? t:f=w999:string)
        n510 = Enqueue Element(queue=w996, element=w999) -> ()  [unwired: 2 in, 3 out]
      }
      event "phoib_release", "phoib_init": Value Change {
        n511 = event-data() -> ()  [unwired: 1 in, 2 out]
        n512 = Flush Queue(queue=w1003) -> (queue out=w1002:refnum<queue>)  [unwired: 1 in, 2 out]
        n513 = Select(t="init" ("name (unnamed)"), s="phoib_init", f="release" ("name (unnamed)")) -> (s? t:f=w1005:string)
        n514 = Enqueue Element(queue=w1002, element=w1005) -> ()  [unwired: 2 in, 3 out]
      }
      event "phoib_standby": Value Change {
        n515 = event-data() -> ()  [unwired: 1 in, 2 out]
        n516 = Enqueue Element(queue=w1009, element="standby") -> ()  [unwired: 2 in, 3 out]
      }
      event "phoib_set": Value Change {
        n517 = event-data() -> ()  [unwired: 1 in, 2 out]
        n518 = Enqueue Element(queue=w1010, element="set") -> ()  [unwired: 2 in, 3 out]
      }
      event "cam_dark": Value Change {
        n519 = event-data() -> ()  [unwired: 1 in, 2 out]
        n520 = Enqueue Element(queue=w1013, element="dark") -> ()  [unwired: 2 in, 3 out]
      }
      event "ROI Left", "ROI Right", "ROI Top", "ROI Bottom", "exposure [ms]", "binning", "gain": Value Change {
        n521 = event-data() -> ()  [unwired: 1 in, 1 out]
        n522 = Enqueue Element(queue=w1015, element="set") -> ()  [unwired: 2 in, 3 out]
      }
      event "cam_saveimg": Value Change {
        n523 = event-data() -> ()  [unwired: 1 in, 1 out]
        n524 = Enqueue Element(queue=w1017, element="single") -> ()  [unwired: 2 in, 3 out]
      }
      event "delscan_go": Value Change {
        n525 = event-data() -> ()  [unwired: 1 in, 1 out]
        n526 = Enqueue Element(queue=w1019, element="GO") -> ()  [unwired: 2 in, 3 out]
      }
      event "delscan_go 2": Value Change {
        n527 = event-data() -> ()  [unwired: 1 in, 1 out]
        n528 = Enqueue Element(queue=w1020, element="delay_chop") -> ()  [unwired: 2 in, 3 out]
      }
      event "Move Abs": Value Change {
        n529 = event-data() -> ()  [unwired: 1 in, 1 out]
      }
      event "ManipRel +", "ManipRel -": Value Change {
        n530 = event-data() -> ()  [unwired: 1 in, 2 out]
        n531 = Negate(x="manip_deltas") -> (-x=w1024:dbl[])
        n532 = Select(t="manip_deltas", s="ManipRel +", f=w1024) -> (s? t:f=w1022:dbl[])
        n533 = Index Array(array=w1022) -> (element #1=w1028:dbl, element #2=w1029:dbl, element #3=w1030:dbl, element #4=w1031:dbl, element #5=w1032:dbl, element #6=w1033:dbl)  [unwired: 6 in]
        n534 = Format Into String(format string="%g_%g_%g_%g_%g_%g", w1028, w1029, w1030, w1031, w1032, w1033) -> (resulting string=w1035:string)  [unwired: 2 in, 1 out]
        n535 = Concatenate Strings("relative:" ("string"), w1035) -> (w1026:string)
        n536 = Enqueue Element(queue=w1036, element=w1026) -> ()  [unwired: 2 in, 3 out]
      }
      event "Optimize": Value Change {
        n537 = event-data() -> ()  [unwired: 1 in, 6 out]
        n538 = Enqueue Element(queue=w1038, element="manip") -> ()  [unwired: 2 in, 3 out]
      }
      event "stop manip": Value Change {
        n539 = event-data() -> ()  [unwired: 1 in, 1 out]
        n540 = Enqueue Element(queue=w1040, element="stop") -> ()  [unwired: 2 in, 3 out]
      }
      event "ESP_go": Value Change {
        w1042 = ":" ("string")
        n541 = event-data() -> ()  [unwired: 1 in, 1 out]
        n542 = local read "ESP Axis"() -> (w1041:i32)
        n543 = Number To Decimal String(number=w1041) -> (decimal integer string=w1044:string)  [unwired: 1 in]
        n544 = Number To Fractional String(number="ESP_dest") -> (F-format string=w1043:string)  [unwired: 3 in]
        n545 = Concatenate Strings("abs:" ("string"), w1044, w1042, w1043, w1042) -> (w1047:string)
        n546 = Enqueue Element(queue=w1048, element=w1047) -> ()  [unwired: 2 in, 3 out]
      }
      event "ESP_set_t0": Value Change {
        n547 = event-data() -> ()  [unwired: 1 in, 1 out]
        n548 = Current VI's Path() -> (path=w1054:path)
        n549 = Strip Path(path=w1054) -> (stripped path=w1050:path)  [unwired: 1 out]
        n550 = Strip Path(path=w1050) -> (stripped path=w1049:path)  [unwired: 1 out]
        n551 = local read "ESP_pos"() -> (w1052:dbl)
        "ESP_t0" <- w1052
        n552 = Number To Fractional String(number=w1052) -> (F-format string=w1051:string)  [unwired: 3 in]
        n553 = Build Path(base path=w1049, name or relative path="t0.txt") -> (appended path=w1053:path)
        n554 = Write to Text File(file (use dialog)=w1053, text=w1051) -> ()  [unwired: 2 in, 3 out]
      }
      event "ESP_+", "ESP_-": Value Change {
        n555 = event-data() -> ()  [unwired: 1 in, 6 out]
        n556 = Negate(x="ESP_delta") -> (-x=w1063:dbl)
        n557 = Select(t="ESP_delta", s="ESP_+", f=w1063) -> (s? t:f=w1061:dbl)
        n558 = Number To Decimal String(number="ESP Axis") -> (decimal integer string=w1058:string)  [unwired: 1 in]
        n559 = Number To Fractional String(number=w1061) -> (F-format string=w1056:string)  [unwired: 3 in]
        n560 = Concatenate Strings("rel:" ("string"), w1058, ":" ("string"), w1056) -> (w1066:string)
        n561 = Enqueue Element(queue=w1060, element=w1066) -> ()  [unwired: 2 in, 3 out]
      }
      event "ESP_dest": Value Change {
        n562 = event-data() -> ()  [unwired: 1 in, 6 out]
        n563 = local read "ESP_dest"() -> (w1070:dbl)
        n564 = local read "ESP_t0"() -> (w1069:dbl)
        n565 = call "mm2time.vi"("fs?"=TRUE ("fs[1]/ps[0]"), "Offset (mm)"=w1069, "distance (mm)"=w1070) -> ("time in fs/ps seconds"=w1067:dbl)
        n566 = local write "ESP_dest_t"(w1067) -> ()
      }
      event "ESP_dest_t": Value Change {
        n567 = event-data() -> ()  [unwired: 1 in, 1 out]
        n568 = local read "ESP_t0"() -> (w1073:dbl)
        n569 = call "time2mm.vi"("fs[1]/ps[0]"=TRUE, "Offset (mm)"=w1073, "time"="ESP_dest_t") -> ("position (mm)"=w1071:dbl)
        n570 = local write "ESP_dest"(w1071) -> ()
      }
      event "load delay table": Value Change {
        n571 = event-data() -> ()  [unwired: 1 in, 6 out]
        n572 = call-poly <vilib>:"Read Delimited Spreadsheet.vi"() -> ("all rows"=w1076:string[][])  [unwired: 10 in, 5 out]
        n573 = local read "binning"() -> (w1083:u16)
        n574 = local write "delay table [fs]"(w1076) -> ()
        n575 = local read "delscan_iters"() -> (w1077:u32)
        n576 = local read "time / step"() -> (w1086:dbl)
        n577 = Array Size(array=w1076) -> (size(s)=w1087:i32[])
        n578 = Index Array(array=dbl[] [8.79, 2.2, 0.553, 0.138], index=w1083) -> (element=w1081:dbl)
        n579 = Index Array(array=w1087) -> (element #1=w1075:i32)  [unwired: 2 in, 1 out]
        n580 = Multiply(x=w1077, y=w1075) -> (x*y=w1080:u32)
        n581 = Multiply(x=w1075, y=w1081) -> (x*y=w1082:dbl)
        n582 = Multiply(x=w1080, y=w1086) -> (x*y=w1085:dbl)
        n583 = Increment(x=w1080) -> (x+1=w1079:u32)
        n584 = Multiply(x=w1079, y=w1081) -> (x*y=w1078:dbl)
        n585 = local write "delaypoints"(w1075) -> ()
        n586 = local write "total steps"(w1080) -> ()
        n587 = local write "duration [HH:MM:SS]"(w1085) -> ()
        n588 = local write "RAM [MB]"(w1082) -> ()
        n589 = local write "disk [MB]"(w1078) -> ()
      }
      event "delay table [fs]", "delscan_iters": Value Change {
        n590 = event-data() -> ()  [unwired: 1 in, 6 out]
        n591 = local read "binning"() -> (w1096:u16)
        n592 = local read "delay table [fs]"() -> (w1100:string[][])
        n593 = local read "delscan_iters"() -> (w1090:u32)
        n594 = local read "time / step"() -> (w1098:dbl)
        n595 = Array Size(array=w1100) -> (size(s)=w1099:i32[])
        n596 = Index Array(array=dbl[] [8.79, 2.2, 0.553, 0.138], index=w1096) -> (element=w1094:dbl)
        n597 = Index Array(array=w1099) -> (element #1=w1088:i32)  [unwired: 2 in, 1 out]
        n598 = Multiply(x=w1090, y=w1088) -> (x*y=w1093:u32)
        n599 = Multiply(x=w1088, y=w1094) -> (x*y=w1095:dbl)
        n600 = Multiply(x=w1093, y=w1098) -> (x*y=w1097:dbl)
        n601 = Increment(x=w1093) -> (x+1=w1092:u32)
        n602 = Multiply(x=w1092, y=w1094) -> (x*y=w1091:dbl)
        n603 = local write "delaypoints"(w1088) -> ()
        n604 = local write "total steps"(w1093) -> ()
        n605 = local write "duration [HH:MM:SS]"(w1097) -> ()
        n606 = local write "RAM [MB]"(w1095) -> ()
        n607 = local write "disk [MB]"(w1091) -> ()
      }
      event "generate delay table": Value Change {
        n608 = event-data() -> ()  [unwired: 1 in, 1 out]
        n609 = call "getdelaypoints.vi"("delscan_stepsize"="delscan_stepsize", "delscan_end"="delscan_end", "delscan_start"="delscan_start") -> ("delaypoints"=w1116:dbl[])
        n610 = Number To Fractional String(number=w1116) -> (F-format string=w1115:string[])  [unwired: 3 in]
        n611 = Build Array(w1115) -> (w1114:string[][])
        n612 = Transpose 2D Array(2D array=w1114) -> (transposed array=w1101:string[][])
        n613 = local write "delay table [fs]"(w1101) -> ()
        n614 = local read "binning"() -> (w1110:u16)
        n615 = local read "delscan_iters"() -> (w1104:u32)
        n616 = local read "time / step"() -> (w1112:dbl)
        n617 = Array Size(array=w1101) -> (size(s)=w1113:i32[])
        n618 = Index Array(array=dbl[] [8.79, 2.2, 0.553, 0.138], index=w1110) -> (element=w1108:dbl)
        n619 = Index Array(array=w1113) -> (element #1=w1102:i32)  [unwired: 2 in, 1 out]
        n620 = Multiply(x=w1104, y=w1102) -> (x*y=w1107:u32)
        n621 = Multiply(x=w1102, y=w1108) -> (x*y=w1109:dbl)
        n622 = Multiply(x=w1107, y=w1112) -> (x*y=w1111:dbl)
        n623 = Increment(x=w1107) -> (x+1=w1106:u32)
        n624 = Multiply(x=w1106, y=w1108) -> (x*y=w1105:dbl)
        n625 = local write "delaypoints"(w1102) -> ()
        n626 = local write "total steps"(w1107) -> ()
        n627 = local write "duration [HH:MM:SS]"(w1111) -> ()
        n628 = local write "RAM [MB]"(w1109) -> ()
        n629 = local write "disk [MB]"(w1105) -> ()
      }
      event "mainimg": Cursor Release {
        n630 = event-data() -> ()  [unwired: 1 in, 1 out]
        n631 = Enqueue Element(queue=w1121, element="refresh") -> ()  [unwired: 2 in, 3 out]
      }
      event "dev_bench": Value Change {
        n632 = event-data() -> ()  [unwired: 1 in, 2 out]
        n633 = Enqueue Element(queue=w1122, element="bench") -> ()  [unwired: 2 in, 3 out]
      }
    }
  }
  n634 = while {
    tunnel: w13 -> [w1132]
    shift-right: [w1130] -> _
    shift-left: _ -> [w1128]
    shift-right: [w1129] -> _
    shift-left: _ -> [w1127]
    shift-right: [w1125] -> _
    shift-left: 0 -> [w1126]
    tunnel: w2 -> [w1124]
    stop <- w1131 stop-if-true
    # "ESP"
    n635 = Preview Queue Element(queue=w1132, timeout in ms (-1)=w1126) -> (queue out=w1135:refnum<queue>, element=w1136:string)  [unwired: 1 in, 2 out]
    n636 = Match Pattern(string=w1136, regular expression=":") -> (before substring=w1134:string, after substring=w1133:string)  [unwired: 1 in, 2 out]
    n637 = case shown="\"init\"" w1134 {
      tunnel: w1135 -> [_ w1147 w1165 w1199 w1200 w1207 w1212]
      tunnel: w1133 -> [_ w1152 w1172 _ _ _ _]
      tunnel: [_ _ _ _ _ TRUE _] -> w1131
      tunnel: [w1139 w1154 w1166 w1197 refnum<visa-resource-name> refnum ("VISA resource name out") w1204 w1211] -> w1130
      tunnel: [w1138 w1155 w1164 w1196 w1202 w1205 w1210] -> w1129
      tunnel: w1128 -> [w1143 w1157 w1170 w1197 w1203 w1204 _]
      tunnel: w1127 -> [w1142 w1156 w1171 w1196 _ w1205 _]
      tunnel: [_ _ _ -1 _ _ _] -> w1125
      tunnel: w1124 -> [_ _ w1163 _ _ _ _]
      frame "idle", Default {
        n638 = local read "ESP Axis"() -> (w1140:i32)
        n639 = local read "ESP_t0"() -> (w1146:dbl)
        n640 = call "Read Actual Position.vi"("error in (no error)"=w1142, "Axis (1)"=w1140, "VISA resource name"=w1143) -> ("error out"=w1138:errorcluster, "Position (units)"=w1141:dbl, "VISA resource name out"=w1139:refnum<visa-resource-name>)  [unwired: 2 in]
        "ESP_pos" <- w1141
        n641 = call "mm2time.vi"("fs?"=TRUE, "Offset (mm)"=w1146, "distance (mm)"=w1141) -> ("time in fs/ps seconds"=→"ESP_delay":dbl)
      }
      frame "rel" {
        n642 = Match Pattern(string=w1152, regular expression=":") -> (before substring=w1151:string, after substring=w1150:string)  [unwired: 1 in, 2 out]
        n643 = Dequeue Element(queue=w1147) -> ()  [unwired: 2 in, 4 out]
        n644 = Decimal String To Number(string=w1151) -> (number=w1149:i32)  [unwired: 2 in, 1 out]
        n645 = Fract/Exp String To Number(string=w1150) -> (number=w1148:dbl)  [unwired: 3 in, 1 out]
        n646 = call "Move Relative.vi"("error in (no error)"=w1156, "Position (0 units)"=w1148, "Axis (1)"=w1149, "VISA resource name"=w1157) -> ("error out"=w1155:errorcluster, "VISA resource name out"=w1154:refnum<visa-resource-name>)  [unwired: 2 in]
      }
      frame "abs" {
        n647 = Dequeue Element(queue=w1165) -> ()  [unwired: 2 in, 4 out]
        n648 = Match Pattern(string=w1172, regular expression=":") -> (before substring=w1173:string, after substring=w1161:string)  [unwired: 1 in, 2 out]
        n649 = Match Pattern(string=w1161, regular expression=":") -> (before substring=w1160:string, after substring=w1159:string)  [unwired: 1 in, 2 out]
        n650 = Decimal String To Number(string=w1173) -> (number=w1169:i32)  [unwired: 2 in, 1 out]
        n651 = Fract/Exp String To Number(string=w1160) -> (number=w1158:dbl)  [unwired: 3 in, 1 out]
        n652 = call "Move Absolute.vi"("error in (no error)"=w1171, "Position (0 units)"=w1158, "Axis (1)"=w1169, "VISA resource name"=w1170) -> ("error out"=w1167:errorcluster, "VISA resource name out"=w1168:refnum<visa-resource-name>)  [unwired: 2 in]
        n653 = case shown="\"wait\"" w1159 {
          tunnel: w1169 -> [_ w1181]
          tunnel: w1168 -> [w1176 w1186]
          tunnel: w1167 -> [w1175 w1185]
          tunnel: [w1176 w1178] -> w1166
          tunnel: [w1175 w1184] -> w1164
          tunnel: w1163 -> [_ w1183]
          frame "", Default {
          }
          frame "wait" {
            n654 = while {
              tunnel: w1181 -> [w1195]
              shift-right: [w1192] -> w1180
              shift-left: w1186 -> [w1194]
              shift-right: [w1191] -> w1179
              shift-left: w1185 -> [w1193]
              stop <- w1190 stop-if-true
              n655 = call "Get Axis Motion Status.vi"("error in (no error)"=w1193, "Axis (1)"=w1195, "VISA resource name"=w1194) -> ("error out"=w1191:errorcluster, "Motion Done"=w1190:bool, "VISA resource name out"=w1192:refnum<visa-resource-name>)  [unwired: 2 in]
            }
            n656 = flat-sequence {
              tunnel: w1180 -> [w1189]
              tunnel: w1179 -> [w1188]
              tunnel: [w1189] -> w1178
              tunnel: [w1188] -> w1177
              frame #0 {
                n657 = Wait (ms)(milliseconds to wait=u32 1000) -> ()  [unwired: 1 out]
              }
            }
            n658 = Enqueue Element(queue=w1183, element="done", error in (no error)=w1177) -> (error out=w1184:errorcluster)  [unwired: 1 in, 2 out]
          }
        }
      }
      frame "suspend" {
        n659 = Dequeue Element(queue=w1199) -> ()  [unwired: 2 in, 4 out]
      }
      frame "release" {
        n660 = Dequeue Element(queue=w1200) -> ()  [unwired: 2 in, 4 out]
        n661 = call "Close.vi"("VISA resource name"=w1203) -> ("error out"=w1202:errorcluster)  [unwired: 10 in]
      }
      frame "close" {
        n662 = Release Queue(queue=w1207) -> ()  [unwired: 2 in, 3 out]
      }
      frame "init" {
        n663 = Dequeue Element(queue=w1212) -> ()  [unwired: 2 in, 4 out]
        n664 = flat-sequence {
          tunnel: [w1215] -> w1209
          tunnel: [w1214] -> w1208
          tunnel: [w1219] -> w1210
          tunnel: [w1220] -> w1211
          tunnel: w1209 -> [w1220]
          tunnel: w1208 -> [w1219]
          frame #0 {
            n665 = local write "ESP_con?"(FALSE ("ESP_con?")) -> ()
          }
          frame #1 {
            n666 = call "Initialize.vi"("VISA resource name"="ESP301 VISA", "Serial Link (RS232)"=enum16{"RS232", "USB"}."USB") -> ("VISA resource name out"=w1215:refnum<visa-resource-name>, "error out"=w1214:errorcluster)  [unwired: 7 in]
          }
          frame #2 {
            n667 = local write "ESP_con?"(TRUE ("ESP_con?")) -> ()
          }
        }
      }
    }
    "error out" <- w1129
  }
  n668 = while {
    tunnel: w3 -> [w1229]
    shift-right: [w1227] -> _
    shift-left: _ -> [w1225]
    shift-right: [w1226] -> _
    shift-left: _ -> [w1224]
    shift-right: [w1222] -> _
    shift-left: 0 -> [w1223]
    tunnel: w2 -> [w1221]
    stop <- w1228 stop-if-true
    # "manip"
    n669 = Preview Queue Element(queue=w1229, timeout in ms (-1)=w1223) -> (queue out=w1232:refnum<queue>, element=w1233:string)  [unwired: 1 in, 2 out]
    n670 = Match Pattern(string=w1233, regular expression=":") -> (before substring=w1231:string, after substring=w1230:string)  [unwired: 1 in, 2 out]
    n671 = case shown="\"init\"" w1231 {
      tunnel: w1232 -> [_ w1245 w1272 w1299 w1303 w1312 w1317]
      tunnel: w1230 -> [_ _ w1259 _ _ _ _]
      tunnel: [_ _ _ _ _ TRUE _] -> w1228
      tunnel: [w1239 w1247 w1251 w1301 refnum<k5> refnum ("gateway_connection out") w1310 w1316] -> w1227
      tunnel: [w1238 w1246 w1253 w1300 w1305 w1309 w1315] -> w1226
      tunnel: w1225 -> [w1241 w1249 w1275 w1301 w1307 w1310 _]
      tunnel: w1224 -> [w1240 w1248 w1274 w1300 _ w1309 _]
      tunnel: [_ _ _ -1 _ _ _] -> w1222
      tunnel: w1221 -> [_ _ w1250 _ _ _ _]
      frame "idle", Default {
        n672 = call "sp_manip_get_axis_status.vi"("error in"=w1240, "gateway_connection"=w1241) -> ("error out"=w1238:errorcluster, "axis_out"=w1237:T9, "gateway_connection out"=w1239:refnum<k5>)  [unwired: 5 in, 2 out]
        n673 = for {
          tunnel: w1237 -> [w1244] mode=indexing
          tunnel: [w1243] -> w1236 mode=indexing
          tunnel: [w1242] -> w1235 mode=indexing
          n674 = Unbundle By Name(w1244) -> ("Axis_Position"=w1243:dbl, "moving"=w1242:bool)
        }
        "moving?" <- w1235
        n675 = local write "pos"(w1236) -> ()
      }
      frame "stop" {
        n676 = Dequeue Element(queue=w1245) -> ()  [unwired: 2 in, 4 out]
        n677 = call "sp_manip_abort.vi"("error in"=w1248, "gateway_connection"=w1249) -> ("error out"=w1246:errorcluster, "gateway_connection out"=w1247:refnum<k5>)  [unwired: 6 in, 2 out]
      }
      frame "relative" {
        n678 = Dequeue Element(queue=w1272) -> ()  [unwired: 2 in, 4 out]
        n679 = Match Pattern(string=w1259, regular expression=":") -> (before substring=w1258:string, after substring=w1257:string)  [unwired: 1 in, 2 out]
        n680 = Equal?(x=w1257, y="wait") -> (x = y?=w1255:bool)
        n681 = call "sp_manip_get_axis_status.vi"("error in"=w1274, "gateway_connection"=w1275) -> ("error out"=w1277:errorcluster, "axis_out"=w1264:T9, "gateway_connection out"=w1276:refnum<k5>)  [unwired: 5 in, 2 out]
        n682 = Scan From String(format string="%g_%g_%g_%g_%g_%g", input string=w1258) -> (output 1=w1271:dbl, output 2=w1270:dbl, output 3=w1269:dbl, output 4=w1268:dbl, output 5=w1267:dbl, output 6=w1266:dbl)  [unwired: 8 in, 3 out]
        n683 = for {
          tunnel: w1264 -> [w1298] mode=indexing
          tunnel: [w1297] -> w1262 mode=indexing
          tunnel: [w1296] -> w1263 mode=indexing
          n684 = Unbundle By Name(w1298) -> ("Axis_Name"=w1297:string, "Axis_Position"=w1296:dbl)
        }
        n685 = Build Array(w1271, w1270, w1269, w1268, w1267, w1266) -> (w1265:dbl[])
        n686 = Add(x=w1263, y=w1265) -> (x+y=w1261:dbl[])
        n687 = call "sp_manip_start_move.vi"("error in"=w1277, "target positions"=w1261, "axis names"=w1262, "gateway_connection"=w1276) -> ("error out"=w1254:errorcluster, "gateway_connection out"=w1252:refnum<k5>)  [unwired: 4 in, 2 out]
        n688 = case shown="True" w1255 {
          tunnel: w1254 -> [w1278 w1285]
          tunnel: [w1278 w1281] -> w1253
          tunnel: w1252 -> [w1279 w1286]
          tunnel: [w1279 w1284] -> w1251
          tunnel: w1250 -> [_ w1280]
          frame False {
          }
          frame True {
            n689 = while {
              tunnel: w1286 -> [w1290]
              tunnel: w1285 -> [w1289]
              tunnel: [w1288] -> w1284
              tunnel: [w1287] -> w1282
              stop <- w1291 continue-if-true
              n690 = call "sp_manip_get_axis_status.vi"("error in"=w1289, "gateway_connection"=w1290) -> ("error out"=w1287:errorcluster, "axis_out"=w1293:T9, "gateway_connection out"=w1288:refnum<k5>)  [unwired: 5 in, 2 out]
              n691 = for {
                tunnel: w1293 -> [w1295] mode=indexing
                tunnel: [w1294] -> w1292 mode=indexing
                n692 = Unbundle By Name(w1295) -> ("moving"=w1294:bool)
              }
              n693 = Or Array Elements(Boolean array=w1292) -> (logical OR=w1291:bool)
            }
            n694 = Enqueue Element(queue=w1280, element="done", error in (no error)=w1282) -> (error out=w1281:errorcluster)  [unwired: 1 in, 2 out]
          }
        }
      }
      frame "suspend" {
        n695 = Dequeue Element(queue=w1299) -> ()  [unwired: 2 in, 4 out]
      }
      frame "release" {
        n696 = Dequeue Element(queue=w1303) -> ()  [unwired: 2 in, 4 out]
        n697 = call "sp_manip_disconnect.vi"("gateway_connection"=w1307) -> ("error out"=w1306:errorcluster, "gateway_connection_out"=w1308:refnum<k5>)  [unwired: 7 in, 2 out]
        n698 = call "tcp_gateway_close_connection.vi"("error in"=w1306, "server_connection"=w1308) -> ("error out"=w1305:errorcluster)  [unwired: 5 in]
      }
      frame "close" {
        n699 = Release Queue(queue=w1312) -> ()  [unwired: 2 in, 3 out]
      }
      frame "init" {
        n700 = Dequeue Element(queue=w1317) -> ()  [unwired: 2 in, 4 out]
        n701 = flat-sequence {
          tunnel: [w1320] -> w1314
          tunnel: [w1319] -> w1313
          tunnel: [w1330] -> w1315
          tunnel: [w1331] -> w1316
          tunnel: w1314 -> [w1331]
          tunnel: w1313 -> [w1330]
          frame #0 {
            n702 = local write "manip_con?"(FALSE ("manip_con?")) -> ()
          }
          frame #1 {
            n703 = call "tcp_gateway_open_connection.vi"() -> ("gateway_connection"=w1323:refnum<k5>, "error out"=w1322:errorcluster)  [unwired: 5 in, 3 out]
            n704 = call "sp_manip_connect.vi"("error in"=w1322, "gateway_connection"=w1323) -> ("error out"=w1319:errorcluster, "axis_out"=w1321:T9, "gateway_connection out"=w1320:refnum<k5>)  [unwired: 5 in, 2 out]
            n705 = for {
              tunnel: w1321 -> [w1328] mode=indexing
              tunnel: [w1327] -> w1324 mode=indexing
              tunnel: [w1326] -> w1325 mode=indexing
              n706 = Unbundle By Name(w1328) -> ("Axis_Name"=w1327:string, "Axis_Position"=w1326:dbl)
            }
            "axis" <- w1324
            "pos" <- w1325
            n707 = local write "dest"(w1325) -> ()
          }
          frame #2 {
            n708 = local write "manip_con?"(TRUE ("manip_con?")) -> ()
          }
        }
      }
    }
    "error out 2" <- w1226
  }
  n709 = while {
    tunnel: w24 -> [w1342]
    shift-right: [w1339] -> _
    shift-left: 0 -> [w1340]
    shift-right: [w1338] -> _
    shift-left: _ -> [w1337]
    shift-right: [w1336] -> _
    shift-left: _ -> [w1335]
    shift-right: [w1334] -> _
    shift-left: u32 0 ("pHandle") -> [w1333]
    tunnel: string[] ["Kinetic Energy", "Pass Energy", "Coil Current", "Work Function", "Detector Voltage", "Screen Voltage", "Conversion Voltage", "Focus Displacement 1", "Focus Displacement 2"] -> [w1332]
    stop <- w1341 stop-if-true
    # "phoib"
    n710 = Preview Queue Element(queue=w1342, timeout in ms (-1)=w1340) -> (queue out=w1345:refnum<queue>, element=w1346:string)  [unwired: 1 in, 2 out]
    n711 = Match Pattern(string=w1346, regular expression=":") -> (before substring=w1344:string, after substring=w1343:string)  [unwired: 1 in, 2 out]
    n712 = case shown="\"standby\"" w1344 {
      tunnel: w1345 -> [_ w1399 w1415 w1431 w1445 w1449 w1455]
      tunnel: w1343 -> [_ _ _ _ _ _ _]
      tunnel: [_ _ _ _ TRUE _ _] -> w1341
      tunnel: [_ _ _ _ _ -1 _] -> w1339
      tunnel: [w1356 w1401 w1418 w1429 w1443 w1448 w1452] -> w1338
      tunnel: w1337 -> [w1367 w1390 w1420 w1430 w1443 w1448 _]
      tunnel: [w1355 w1400 w1417 w1428 w1441 w1446 w1451] -> w1336
      tunnel: w1335 -> [w1365 w1389 w1419 _ w1441 w1446 _]
      tunnel: [w1353 w1387 w1416 w1427 w1442 w1447 w1454] -> w1334
      tunnel: w1333 -> [w1353 w1387 w1416 w1426 w1442 w1447 _]
      tunnel: w1332 -> [w1354 w1380 _ _ _ _ _]
      frame "idle", Default {
        n713 = call "SL2_AD_DLL_Phoibos_GetDeviceState.vi"("dll_path"=w1367, "pHandle_in"=w1353, "dev_type"=DEF_dev_type."devA (analyzer)", "error in"=w1365) -> ("path out"=w1352:path, "state"=→"state":T4, "error out"=w1351:errorcluster)  [unwired: 2 in]
        n714 = for {
          tunnel: w1353 -> [w1374]
          tunnel: w1354 -> [w1372] mode=indexing
          tunnel: [w1371] -> w1364 mode=indexing
          tunnel: [w1370] -> w1356
          shift-right: [w1369] -> w1355
          shift-left: w1351 -> [w1373]
          tunnel: w1352 -> [w1368]
          n715 = call "SL2_AD_DLL_Phoibos_GetVoltage.vi"("error in"=w1373, "voltage_name"=w1372, "pHandle"=w1374, "dll path in"=w1368) -> ("error out"=w1369:errorcluster, "value"=w1371:dbl, "dll path out"=w1370:path)  [unwired: 3 in]
        }
        n716 = Index Array(array=w1364) -> (element #1=→"phoib_I_1":dbl, element #2=→"phoib_I_2":dbl, element #3=→"phoib_I_3":dbl, element #4=→"phoib_I_4":dbl, element #5=→"phoib_I_5":dbl, element #6=→"phoib_I_6":dbl, element #7=→"phoib_I_7":dbl, element #8=→"phoib_I_8":dbl, element #9=→"phoib_I_9":dbl)  [unwired: 9 in]
      }
      frame "set" {
        n717 = Dequeue Element(queue=w1399) -> ()  [unwired: 2 in, 4 out]
        n718 = Multiply(x="VoltageRange", y=13) -> (x*y=w1396:i32)
        n719 = Add(x="Mode", y=w1396) -> (x+y=w1393:i32)
        n720 = Index Array(array=u32[] [251749632, 251749633, 251749634, 251749635, 251749636, 251749637, 251749638, 251749639, 251749640, 251749641, 251749642, 251749643, 251749644, 251749645, 251749646, 251749647, 251749648, 251749649, 251749650, 251749651, 251749652, 251749653, 251749654, 251749655, 251749656, 251749657, 251749658, 251749659, 251749660, 251749661, 251749662, 251749663, 251749664, 251749665, 251749666, 251749667, 251749668, 251749669, 251749670, 251749671, 251749672, 251749673, 251749674, 251749675, 251749676, 251749677, 251749678, 251749679, 251749680, 251749681, 251749682, 251749683, 251749684, 251749685, 251749686, 251749687, 251749688, 251749689, 251749690, 251749691, 251749692, 251749693, 251749694, 251749695, 251749696] ("modeIDs"), index=w1393) -> (element=w1391:u32)
        n721 = Build Array("phoib_I_1s", "phoib_I_2s", "phoib_I_3s", "phoib_I_4s", "phoib_I_5s", "phoib_I_6s", "phoib_I_7s", "phoib_I_8s", "phoib_I_9s") -> (w1379:dbl[])
        n722 = call "SL2_AD_DLL_Phoibos_SetDeviceMode.vi"("pHandle"=w1387, "error in"=w1389, "value"=w1391, "dev_type"=DEF_dev_type."devA (analyzer)", "dll path in"=w1390) -> ("error out"=w1378:errorcluster, "dll path out"=w1388:path)  [unwired: 4 in]
        n723 = for {
          tunnel: w1387 -> [w1407]
          shift-right: [w1414] -> w1401
          shift-left: w1388 -> [w1411]
          tunnel: w1380 -> [w1406] mode=indexing
          tunnel: w1379 -> [w1405] mode=indexing
          shift-right: [w1413] -> w1400
          shift-left: w1378 -> [w1409]
          n724 = call "SL2_AD_DLL_Phoibos_GetVoltageRange.vi"("error in"=w1409, "voltage_name"=w1406, "pHandle"=w1407, "dll path in"=w1411) -> ("error out"=w1408:errorcluster, "min"=w1403:dbl, "max"=w1404:dbl, "dll path out"=w1410:path)  [unwired: 2 in]
          n725 = In Range and Coerce(upper limit=w1404, x=w1405, lower limit=w1403) -> (coerced(x)=w1402:dbl)  [unwired: 1 out]
          n726 = call "SL2_AD_DLL_Phoibos_SetVoltage.vi"("commit"=TRUE, "pHandle"=w1407, "error in"=w1408, "value"=w1402, "voltageName"=w1406, "dll path in"=w1410) -> ("error out"=w1413:errorcluster, "dll path out"=w1414:path)  [unwired: 3 in]
        }
      }
      frame "standby" {
        w1421 = T4 0 items=["Off"=-1, "Standby"=0, "On"=1] ("state")
        n727 = Dequeue Element(queue=w1415) -> ()  [unwired: 2 in, 4 out]
        n728 = call "SL2_AD_DLL_Phoibos_SetDeviceState.vi"("pHandle_in"=w1416, "error in"=w1419, "state"=w1421, "dev_type"=DEF_dev_type."devA (analyzer)", "dll_path"=w1420) -> ("error out"=w1417:errorcluster, "path out"=w1418:path)  [unwired: 2 in]
      }
      frame "release" {
        n729 = Dequeue Element(queue=w1431) -> ()  [unwired: 2 in, 4 out]
        n730 = flat-sequence {
          tunnel: w1430 -> [w1432]
          tunnel: w1426 -> [w1433]
          tunnel: [w1436] -> w1425
          tunnel: [w1435] -> w1424
          tunnel: [u32 0] -> w1423
          tunnel: [w1438] -> w1427
          tunnel: [w1439] -> w1428
          tunnel: [w1440] -> w1429
          tunnel: w1425 -> [w1440]
          tunnel: w1424 -> [w1439]
          tunnel: w1423 -> [w1438]
          frame #0 {
            n731 = call "SL2_AD_DLL_Phoibos_Shutdown.vi"("pHandle"=w1433, "dll path in"=w1432) -> ("error out"=w1435:errorcluster, "dll path out"=w1436:path)  [unwired: 4 in]
          }
          frame #1 {
            n732 = local write "phoib_con?"(FALSE ("phoib_con?")) -> ()
          }
        }
      }
      frame "close" {
        n733 = Release Queue(queue=w1445) -> ()  [unwired: 2 in, 3 out]
      }
      frame "suspend" {
        n734 = Dequeue Element(queue=w1449) -> ()  [unwired: 2 in, 4 out]
      }
      frame "init" {
        n735 = Dequeue Element(queue=w1455) -> ()  [unwired: 2 in, 4 out]
        n736 = flat-sequence {
          tunnel: [w1462] -> w1453
          tunnel: [w1458] -> w1452
          tunnel: [w1457] -> w1451
          tunnel: [w1470] -> w1454
          tunnel: w1453 -> [w1470]
          frame #0 {
            n737 = local write "phoib_con?"(FALSE ("phoib_con?")) -> ()
          }
          frame #1 {
            w1461 = DEF_dev_type."devA (analyzer)" ("dev_type")
            n738 = call "GetSL2AD_VI_dllPath.vi"() -> ("error"=w1465:errorcluster, "Path"=w1466:path)  [unwired: 9 in, 1 out]
            n739 = call "SL2_AD_DLL_List_Devices.vi"("error in"=w1465, "dev_type"=w1461, "dll path in"=w1466) -> ("error out"=w1459:errorcluster, "devices"=w1468:string[], "dll path out"=w1460:path)  [unwired: 2 in]
            n740 = Index Array(array=w1468) -> (element=w1467:string)  [unwired: 1 in]
            n741 = call "SL2_AD_DLL_Phoibos_Initialize.vi"("error in"=w1459, "analyzerId"=w1467, "dll_path"=w1460) -> ("error out"=w1463:errorcluster, "pHandle"=w1462:u32, "path out"=w1464:path)  [unwired: 2 in]
            n742 = call "SL2_AD_DLL_Phoibos_ListDeviceModes.vi"("dll path in"=w1464, "dev_type"=w1461, "pHandle"=w1462, "error in"=w1463) -> ("dll path out"=w1458:path, "error out"=w1457:errorcluster)  [unwired: 1 in, 2 out]
          }
          frame #2 {
            n743 = local write "phoib_con?"(TRUE ("phoib_con?")) -> ()
          }
        }
      }
    }
    "phoib_error" <- w1336
  }
